vi "G#Debugger_CloneUI.vi"(1 "RootClass":string) -> ()   [LabVIEW 2017, in "G#Debugger.lvlib"]
doc: "Debugger for G# Objects."
uses:
  <vilib>/addons/_AddQ/G#Debugger/G#Debugger.lvlib
  <vilib>/addons/_AddQ/G#Debugger/private/G#Debugger_SubPanelInfo.ctl
  <vilib>/addons/_AddQ/G#Object/G#Object.lvclass
  <vilib>/addons/_AddQ/G#Object/utils/G#Object_ClassHierarchy.ctl
  <vilib>/addons/_AddQ/G#Debugger/private/G#Debugger_TreeElement.ctl
  <vilib>/addons/_AddQ/G#Debugger/private/G#Debugger_DebugDialog.vi
  <vilib>/Platform/browser.llb/Open URL in Default Browser (string).vi
panel:
  in  "AggregatorsTags":i32(listbox)
  in  "Help":bool
  out "Application Instance":string
  in  "Window Behaviour":bool
  in  "Window Transparency":u8(slide) max=75 scale=0.0..75.0
  in  "External Create Process Running":bool
  in  "Tab Control":enum32{"Objects", "Trace", "Active Debug"}(tab)
  out "RootCls":string caption="Root Class"
  in  "Aggregators":i32(listbox)
  in  "AggregatesTags":i32(listbox)
  in  "Aggregates":i32(listbox)
  in  "Highlight Aggregates?":bool=TRUE
  in  "Attributes":bool
  in  "Inheritance":i32(listbox)
  in  "Destroy":bool
  in  "ObjectTree":string(tree) caption="Object Tree"
  in  "Refresh":bool
  out "# of Users":i32
  out "Counter":bool
  out "Object Name":string
  out "Full Class Name":string
  in  "Poll Time (ms)":i32=200 min=0
  in  "Garbage collect":bool
  out "Object ID":u32 format="%x"
  in  "Hide Empty Classes?":bool=TRUE
  out "Owner":string
  out "Connected?":bool
  in  "ShowAggregators":bool
  out "To String":string
  in  "Filter Expression":string
  in  "Trace Direction":bool=TRUE
  in  "Clear":bool
  in  "Save":bool
  out "Trace":string
  in  "Max Lines":u32=1000
  out "Run State":string
  out "CachedObjId":u32 caption="Object ID" format="%x"
  in  "Abort VI":bool
  in  "Run VI":bool
  in  "Open Panel":bool
  in  "DebugTree":string(tree)
  in  "Enable Active Debug":bool
  out "Icon":picture
  out "Cached Ref Valid":bool
  in  "Wait Until Done":bool=TRUE
  out "Cached Reference Class Name":string
  out "G# Version":string
  # "G# Clone Debugger"
  # "< Poll to update >"
  # "These logs will also always appear in the NI LabVIEW Desktop Execution Trace, even without debugger running."
  # "The last created reference is automatically cashed and copied to all the new selected , opened or executed methods 'reference in'."
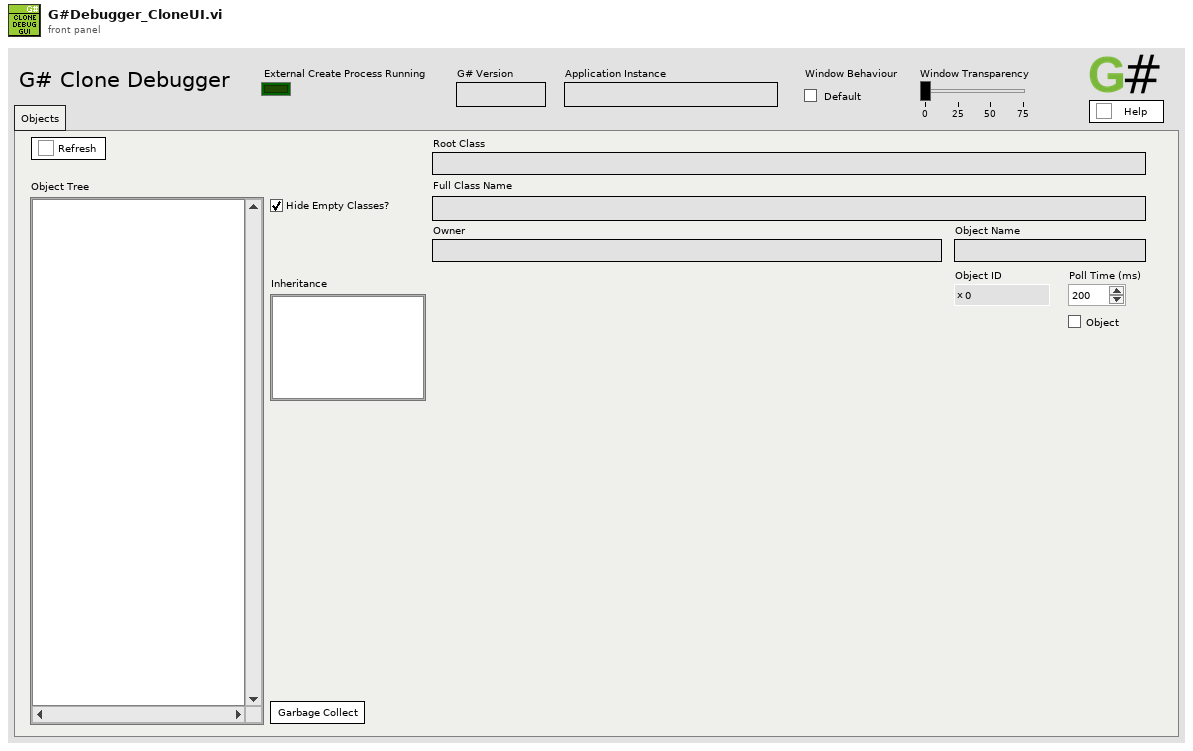
[diagram p1: front panel]
types:
  T1 = cluster{"ObjectName":string, "ObjectID":u32, "Users":i32, "Counter":bool, "AttributeRefs":u32[], "FullClassName":string, "ClassName":string, "Create method":enum16{"Create", "Create or look up existing", "Look up existing"}, "GenericDestructorExists":bool, "Owner":string}[]
  T2 = cluster{"Path":path, "ClsNames":string[], "ClsPaths":path[], "ParPaths":path[]}
  T3 = cluster{"ClassInfoDvr":refnum<data-value>, "sub panel dvr":refnum<data-value>, "CloneUIevent":refnum<user-event>, "Active Project":refnum<vi>, "Front Panel":refnum<vi>}
  T4 = typedef "G#Debugger.lvlib/G#Debugger_SubPanelInfo.ctl" = cluster{"Ref":refnum<class "G#Object.lvclass">, "class hierarchy":T5[], "class attributes":path[], "object attributes":path[], "inheritance index":i32, "is class attributes":bool, "vi reference":refnum<vi>}
  T5 = typedef "G#Object.lvclass/G#Object_ClassHierarchy.ctl" = cluster{"ClassName":string, "FullClassName":string, "ClassPath":path, "IsLeaf":bool}
  T6 = enum8{"Enabled", "Disabled", "Disabled and Grayed Out"}
  T7 = typedef "G#Debugger.lvlib/G#Debugger_TreeElement.ctl" = cluster{"Name":string, "Tag":string, "ParentTag":string, "Position":i32}
  T8 = cluster{"ObjectTree":string, "Attributes":bool, "Inheritance":i32}
  T9 = cluster{"Active Item Row Number":i32, "name":string}
  T10 = enum32{"Invalid", "Default", "Floating", "Floating/Auto-Hide", "Modal"}
  T11 = cluster{"ObjectName":string, "ObjectID":u32, "Users":i32, "Counter":bool, "AttributeRefs":u32[], "FullClassName":string, "ClassName":string, "Create method":enum16{"Create", "Create or look up existing", "Look up existing"}, "GenericDestructorExists":bool, "Owner":string}
  T12 = cluster{"ObjectTree":string, bool, "Inheritance":i32}
  T13 = enum32{"Bad", "Idle", "Run top level", "Running"}
  T14 = cluster{"Active Item Row Number":i32, "name":string}[]
  T15 = typedef "imagedata.ctl" = cluster{"image type":i32, "image depth":i32, "image":u8[], "mask":u8[], "colors":u32[], "Rectangle":cluster{"left":i16, "top":i16, "right":i16, "bottom":i16}}
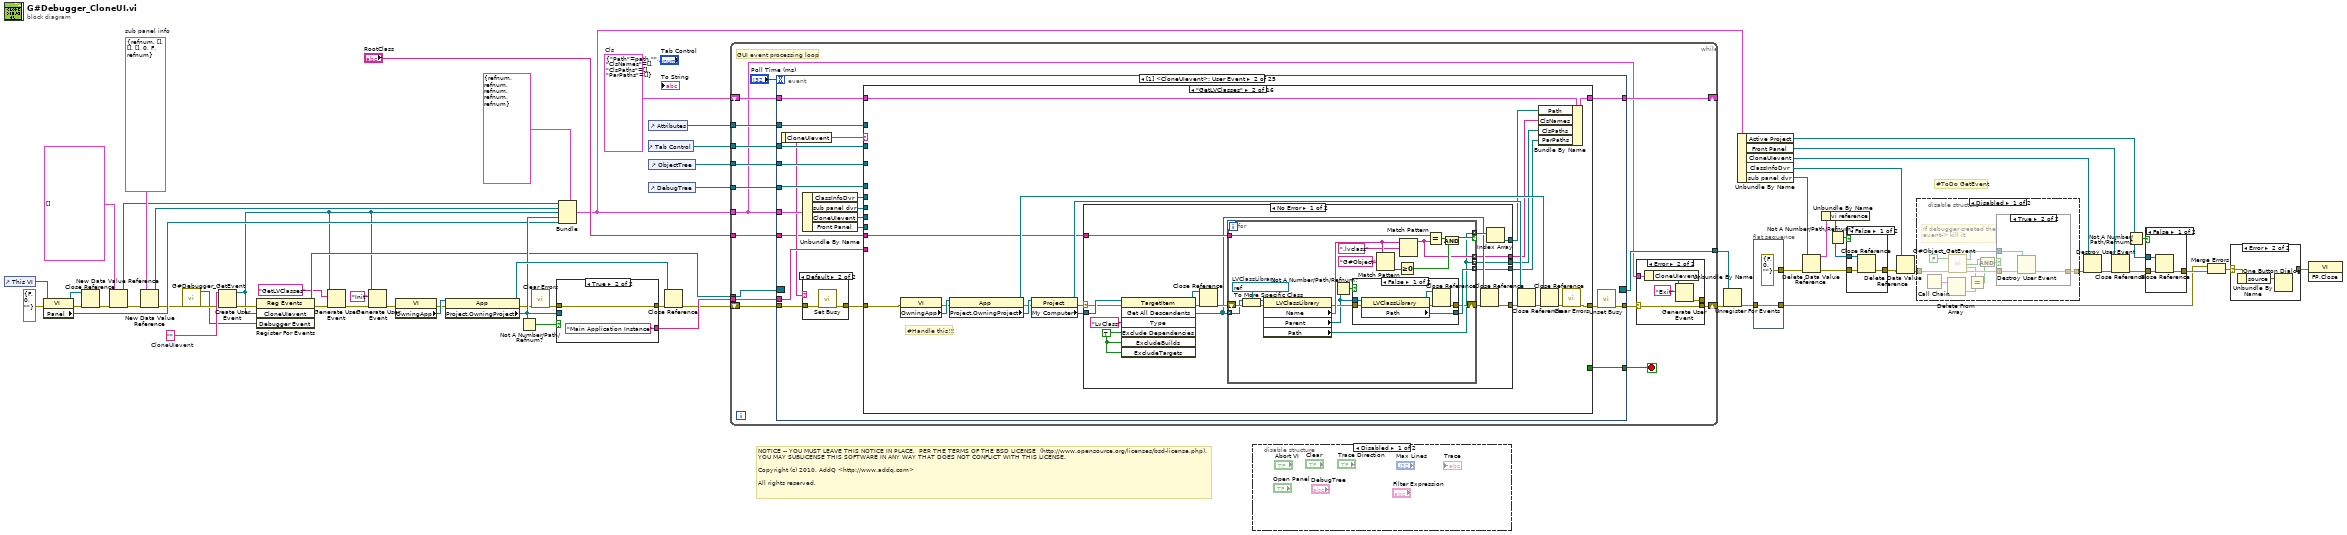
[diagram p0: block diagram]
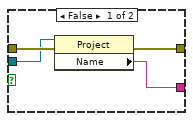
[diagram p7: hidden frame]
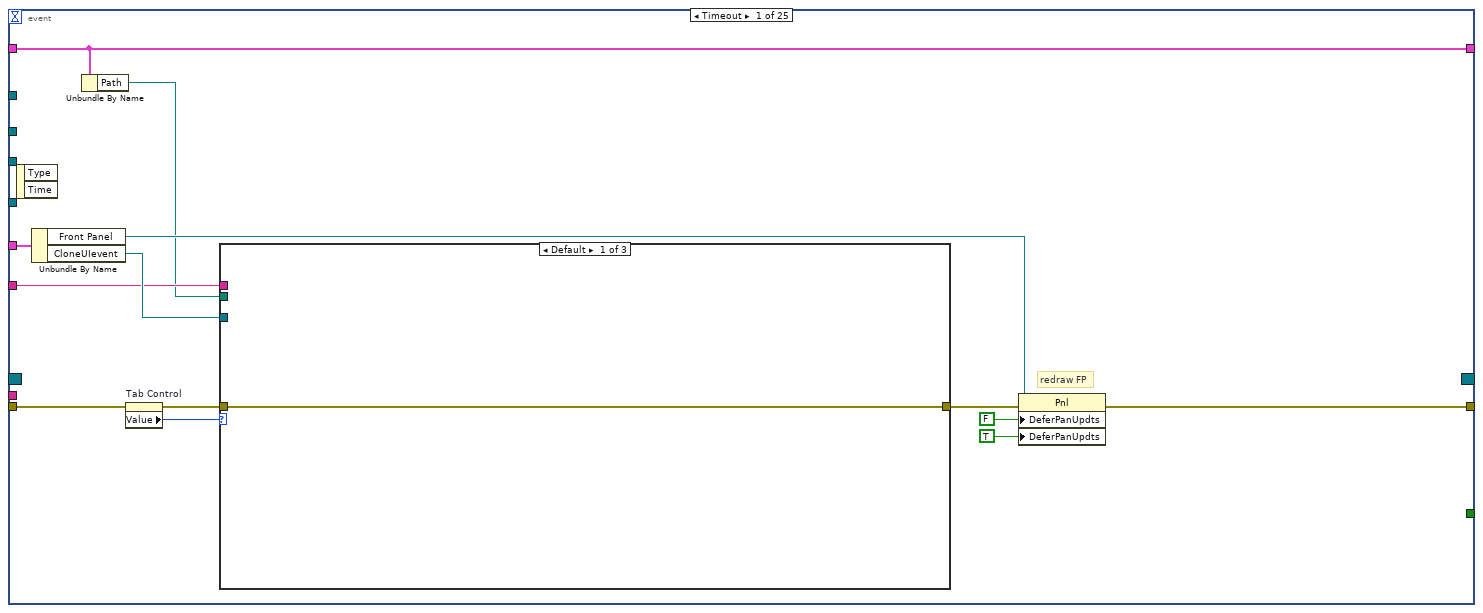
[diagram p10: hidden frame]
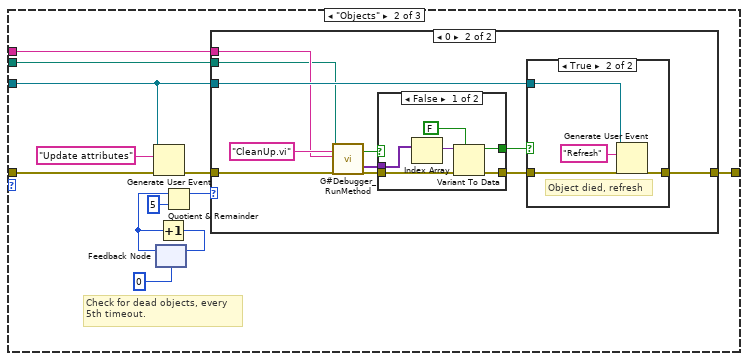
[diagram p11: hidden frame]
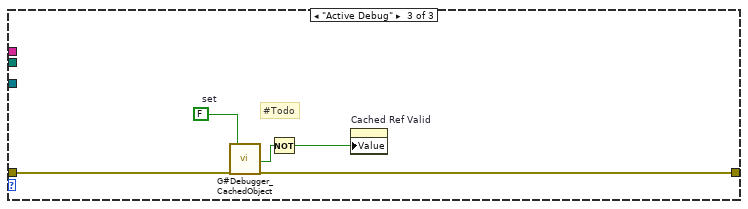
[diagram p15: hidden frame]
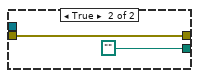
[diagram p18: hidden frame]
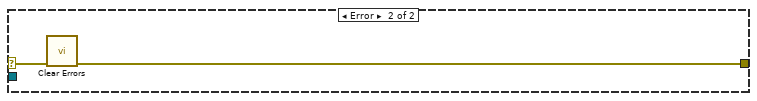
[diagram p19: hidden frame]
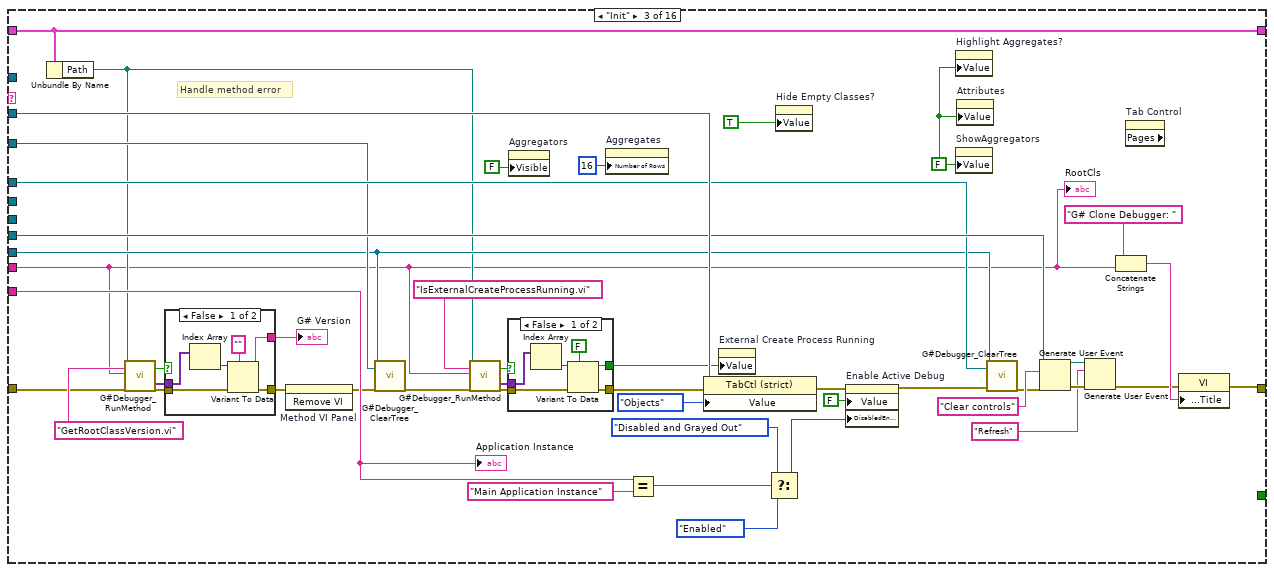
[diagram p20: hidden frame]
diagram:
  w6 = T2 {"Path"=path "", "ClsNames"=[], "ClsPaths"=[], "ParPaths"=[]}  # Cls
  w35 = ""  # CloneUIevent
  w55 = T4 {"Ref"=refnum, "class hierarchy"=[], "class attributes"=[], "object attributes"=[], "inheritance index"=0, "is class attributes"=FALSE, "vi reference"=refnum}  # sub panel info
  # "#ToDo GetEvent"
  # "NOTICE -- YOU MUST LEAVE THIS NOTICE IN PLACE.  PER THE TERMS OF THE BSD LICENSE  (http://www.opensource.org/licenses/bsd-license.php).\nYOU MAY SUBLICENSE THIS SOFTWARE IN ANY WAY THAT DOES NOT CONFLICT WITH THIS LICENSE.\n\nCopyright (c) 2010, AddQ <http://www.addq.com>\n\nAll rights reserved."
  n1 = control-ref of="This VI"() -> (w40:refnum<vi>)
  n2 = property class="VI"(reference=w40, error in=errorcluster {"status"=FALSE, "code"=0, "source"=""} ("error in (no error)")) -> (reference out=w43:refnum<vi>, error out=w44:errorcluster, "Panel"=w42:refnum<vi>)
  n3 = Close Reference(reference=w43, error in (no error)=w44) -> (error out=w41:errorcluster)
  n4 = New Data Value Reference(data value=T1 [], error in=w41) -> (data value reference=w3:refnum<data-value>, error out=w56:errorcluster)
  n5 = New Data Value Reference(data value=w55, error in=w56) -> (data value reference=w54:refnum<data-value>, error out=w34:errorcluster)
  n6 = call <vilib>:"G#Debugger_GetEvent.vi"("error in (no error)"=w34) -> ("Debugger Event"=w32:refnum<user-event>, "error out"=w33:errorcluster)  [unwired: 17 in]
  n7 = Create User Event(user event datatype=w35, error in=w33) -> (user event=w9:refnum<user-event>, error out=w36:errorcluster)
  n8 = register-events(error in=w36, w9, w32) -> (reference out=w39:refnum<event-registration>, error out=w8:errorcluster)  [unwired: 1 in]
  n9 = Generate User Event(user event=w9, event data cluster="GetLVClasses" ("event data"), error in=w8) -> (error out=w7:errorcluster)  [unwired: 1 in, 1 out]
  n10 = Generate User Event(user event=w9, event data cluster="Init" ("event data"), error in=w7) -> (error out=w52:errorcluster)  [unwired: 1 in, 1 out]
  n11 = property class="VI"(error in=w52) -> (error out=w51:errorcluster, "OwningApp"=w53:refnum<vi>)  [unwired: 1 in, 1 out]
  n12 = property class="App"(reference=w53, error in=w51) -> (reference out=w48:refnum<vi>, error out=w46:errorcluster, "Project.OwningProject"=w47:refnum<vi>)
  n13 = Not A Number/Path/Refnum?(number/path/refnum=w47) -> (NaN/Path/Refnum?=w50:bool)
  n14 = call <vilib>:"Clear Errors.vi"("error in (no error)"=w46) -> ("error out"=w45:errorcluster)  [unwired: 5 in, 1 out]
  n15 = case shown="True" w50 {
    tunnel: w45 -> [w68 w70]
    tunnel: w47 -> [w67 _]
    tunnel: [w65 w70] -> w49
    tunnel: [w66 "Main Application Instance" ("Name")] -> w38
    frame False {
      n16 = property class="Project"(reference=w67, error in=w68) -> (error out=w65:errorcluster, "Name"=w66:string)  [unwired: 1 out]
    }
    frame True {
    }
  }
  n17 = Bundle(cluster=T3 {"ClassInfoDvr"=refnum, "sub panel dvr"=refnum, "CloneUIevent"=refnum, "Active Project"=refnum, "Front Panel"=refnum} ("refs"), "ClassInfoDvr"=w3, "sub panel dvr"=w54, "CloneUIevent"=w9, "Active Project"=w47, "Front Panel"=w42) -> (w14:T3)
  n18 = control-ref of="Attributes"() -> (w59:refnum<vi>)
  n19 = control-ref of="Tab Control"() -> (w64:refnum<vi>)
  n20 = control-ref of="ObjectTree"() -> (w60:refnum<vi>)
  n21 = control-ref of="DebugTree"() -> (w63:refnum<vi>)
  n22 = Close Reference(reference=w48, error in (no error)=w49) -> (error out=w37:errorcluster)
  n23 = while {
    shift-right: [w73] -> w62
    shift-left: w37 -> [w82]
    tunnel: w60 -> [w86]
    tunnel: w14 -> [w71]
    tunnel: w64 -> [w84]
    tunnel: w63 -> [w83]
    tunnel: w39 -> [w81]
    tunnel: [w78] -> w61
    tunnel: w38 -> [w79]
    tunnel: w59 -> [w77]
    tunnel: "RootClass" -> [w76]
    shift-right: [w75] -> _
    shift-left: w6 -> [w74]
    stop <- w85 stop-if-true
    # "GUI event processing loop"
    n24 = event shown="[1] <CloneUIevent>: User Event" {
      selector: w81 -> [_ _ _ _ _ _ _ _ _ _ _ _ _ _ _ _ _ _ _ _ _ _ _ _ _]
      dyn-events: [_ _ _ _ _ _ _ _ _ _ _ _ _ _ _ _ _ _ _ _ _ _ _ _ _] -> w78
      timeout: "Poll Time (ms)" -> [_ _ _ _ _ _ _ _ _ _ _ _ _ _ _ _ _ _ _ _ _ _ _ _ _]
      tunnel: w82 -> [w101 w153 w883 w894 w902 w913 w928 w933 w986 w1041 w1063 w1071 w1076 w1084 w1089 w1102 w1131 w1166 w1172 w1222 w1230 w1236 w1250 w1266 w1277]
      tunnel: [w98 w155 w882 w894 w902 w912 w927 w932 w981 w1040 w1062 w1072 w1074 w1082 w1095 w1114 w1129 w1163 w1171 w1221 w1229 w1235 w1250 w1265 w1274] -> w72
      tunnel: w86 -> [_ w166 _ w895 w903 _ _ _ w985 _ _ w1070 _ _ _ _ w1128 _ _ _ _ _ _ _ w1276]
      tunnel: [_ w165 _ _ _ _ FALSE _ _ _ _ _ _ _ _ _ _ _ _ _ _ _ _ _ _] -> w85
      tunnel: w71 -> [w105 w164 w881 _ _ w911 w926 w931 w983 _ w1061 _ w1075 w1083 _ w1112 w1125 _ w1170 _ _ _ _ _ w1273]
      tunnel: w84 -> [_ w161 _ _ _ _ _ _ _ _ _ _ _ _ _ _ _ _ _ _ _ _ _ _ _]
      tunnel: w83 -> [_ w159 _ _ _ _ _ _ _ _ _ _ _ _ _ _ _ _ w1173 _ _ _ _ _ _]
      tunnel: w79 -> [_ w158 _ _ _ _ _ _ _ _ _ _ _ _ _ _ _ _ w1169 _ _ _ _ _ _]
      tunnel: w77 -> [_ w151 _ _ _ _ _ _ _ _ _ _ _ _ _ _ _ _ _ _ _ _ _ _ _]
      tunnel: w76 -> [w95 w150 _ _ _ _ _ _ _ _ _ _ _ _ w1090 w1098 _ _ _ _ _ w1233 _ w1262 _]
      tunnel: [w94 w149 w880 w891 w899 w907 w921 w929 w969 w1030 w1060 w1066 w1073 w1079 w1087 w1106 w1124 w1162 w1167 w1218 w1224 w1232 w1247 w1264 w1272] -> w75
      tunnel: w74 -> [w94 w148 w880 w891 w899 w907 w921 w929 w969 w1030 w1060 w1066 w1073 w1079 w1087 w1106 w1124 w1162 w1167 w1218 w1224 w1232 w1247 w1264 w1272]
      event Timeout {
        # "redraw FP"
        n25 = event-data() -> ()  [unwired: 1 in, 2 out]
        n26 = Unbundle By Name(w105) -> ("Front Panel"=w99:refnum<vi>, "CloneUIevent"=w104:refnum<user-event>)
        n27 = Unbundle By Name(w94) -> ("Path"=w93:path)
        n28 = property on="Tab Control" class="TabCtl (strict)"(error in=w101) -> (error out=w102:errorcluster, "Value"=w103:enum32{"Objects", "Trace", "Active Debug"})  [unwired: 1 in, 1 out]
        n29 = case shown="Default" w103 {
          tunnel: w102 -> [w106 w118 w145]
          tunnel: w104 -> [_ w114 _]
          tunnel: [w106 w115 w144] -> w100
          tunnel: w93 -> [_ w108 _]
          tunnel: w95 -> [_ w107 _]
          frame Default {
          }
          frame "Objects" {
            # "Check for dead objects, every\n5th timeout."
            n30 = Generate User Event(user event=w114, event data cluster="Update attributes" ("event data"), error in=w118) -> (error out=w116:errorcluster)  [unwired: 1 in, 1 out]
            n31 = feedback #1(u64 0) -> (w110:u64)
            n32 = Increment(x=w110) -> (x+1=w109:u64)
            n33 = feedback-in #1(w109) -> ()
            n34 = Quotient & Remainder(x=w110, y=u64 5) -> (x-y*floor(x/y)=w113:u64)  [unwired: 1 out]
            n35 = case shown="0" w113 {
              tunnel: w116 -> [w119 w127]
              tunnel: [w119 w130] -> w115
              tunnel: w114 -> [_ w129]
              tunnel: w108 -> [_ w121]
              tunnel: w107 -> [_ w126]
              frame Default {
              }
              frame 0 {
                n36 = call <vilib>:"G#Debugger_RunMethod.vi"("ClassPath"=w121, "MethodName"="CleanUp.vi" ("name or relative path"), "ClassPrefix"=w126, "error in (no error)"=w127) -> ("Error?"=w120:bool, "ControlValue out"=w125:variant[], "error out"=w124:errorcluster)  [unwired: 13 in]
                n37 = case shown="False" w120 {
                  tunnel: w125 -> [w136 _]
                  tunnel: w124 -> [w135 w137]
                  tunnel: [w132 _] -> w123
                  tunnel: [w131 w137] -> w122
                  frame False {
                    n38 = Index Array(array=w136) -> (element=w133:variant)  [unwired: 1 in]
                    n39 = Variant To Data(error in=w135, type=FALSE, Variant=w133) -> (data=w132:bool, error out=w131:errorcluster)
                  }
                  frame True {
                  }
                }
                n40 = case shown="True" w123 {
                  tunnel: w122 -> [w138 w141]
                  tunnel: [w138 w140] -> w130
                  tunnel: w129 -> [_ w139]
                  frame False {
                  }
                  frame True {
                    # "Object died, refresh"
                    n41 = Generate User Event(user event=w139, event data cluster="Refresh" ("event data"), error in=w141) -> (error out=w140:errorcluster)  [unwired: 1 in, 1 out]
                  }
                }
              }
            }
          }
          frame "Active Debug" {
            w147 = FALSE  # set
            # "#Todo"
            n42 = call <vilib>:"G#Debugger_CachedObject.vi"("error in (no error)"=w145, "set"=w147) -> ("not a refnum?"=w146:bool, "error out"=w144:errorcluster)  [unwired: 15 in, 1 out]
            n43 = Not(x=w146) -> (.not. x?=w143:bool)
            n44 = property on="Cached Ref Valid" class="Bool (strict)"("Value"=w143) -> ()  [unwired: 2 in, 2 out]
          }
        }
        n45 = property class="Pnl"(reference=w99, error in=w100, "DeferPanUpdts"=FALSE ("Defer Panel Updates"), "DeferPanUpdts"=TRUE ("Defer Panel Updates")) -> (error out=w98:errorcluster)  [unwired: 1 out]
      }
      event User Event {
        n46 = event-data() -> ("CloneUIevent"=w154:string)  [unwired: 1 in]
        n47 = Unbundle By Name(w164) -> ("ClassInfoDvr"=w163:refnum<data-value>, "sub panel dvr"=w162:refnum<data-value>, "CloneUIevent"=w160:refnum<user-event>, "Front Panel"=w157:refnum<vi>)
        n48 = case shown="Default" w154 {
          tunnel: w153 -> [w167 w169]
          tunnel: [w167 w168] -> w152
          frame "Clear object tab", "Update attributes" {
          }
          frame Default {
            n49 = call <vilib>:"Set Busy.vi"("error in (no error)"=w169) -> ("error out"=w168:errorcluster)  [unwired: 9 in, 1 out]
          }
        }
        n50 = case shown="\"GetLVClasses\"" w154 {
          selector: w154 -> [_ _ _ _ _ _ _ _ _ _ _ _ w708 _ _ w878]
          tunnel: [w171 w178 w258 w301 w312 w322 w347 w374 w439 w463 w606 w655 w704 w712 w764 w879] -> w156
          tunnel: w152 -> [w171 w180 w250 w302 w312 w321 w337 w376 w441 w458 w609 w656 w704 w716 w768 w879]
          tunnel: [_ _ _ _ _ TRUE _ _ _ _ _ _ _ _ _ _] -> w165
          tunnel: w163 -> [_ _ _ _ _ _ _ w380 w430 w466 _ _ _ w714 w766 _]
          tunnel: w166 -> [_ _ w276 _ _ _ _ w391 w440 w460 w610 _ _ w711 w763 _]
          tunnel: w162 -> [_ _ _ _ _ _ _ _ _ w465 w598 _ _ _ _ _]
          tunnel: w161 -> [_ _ w283 _ _ _ _ _ _ _ _ _ _ _ _ _]
          tunnel: w160 -> [_ _ w281 w300 _ _ w349 w384 w438 w464 _ _ _ _ _ _]
          tunnel: w159 -> [_ _ w277 _ _ _ _ _ _ _ _ _ _ _ _ _]
          tunnel: w158 -> [_ _ w274 _ _ _ _ _ _ _ _ _ _ _ _ _]
          tunnel: w157 -> [_ _ w263 _ _ _ _ w392 w436 _ _ _ _ w710 w762 _]
          tunnel: w151 -> [_ _ _ _ _ _ _ _ _ w461 _ _ _ _ _ _]
          tunnel: w150 -> [_ w179 w239 _ _ w318 w339 w370 w429 _ w604 _ _ _ _ _]
          tunnel: [w170 w172 w245 w298 w307 w317 w350 w383 w427 w459 w612 w654 w703 w709 w761 w875] -> w149
          tunnel: w148 -> [w170 w177 w245 w298 w307 w317 w350 w383 w427 w459 w612 w654 w703 w709 w761 w875]
          frame Default {
          }
          frame "GetLVClasses" {
            # "#Handle this!!!"
            n51 = property class="VI"(error in=w180) -> (error out=w190:errorcluster, "OwningApp"=w191:refnum<vi>)  [unwired: 1 in, 1 out]
            n52 = property class="App"(reference=w191, error in=w190) -> (reference out=w189:refnum<vi>, error out=w183:errorcluster, "Project.OwningProject"=w184:refnum<vi>)
            n53 = property class="Project"(reference=w184, error in=w183) -> (reference out=w188:refnum<vi>, error out=w186:errorcluster, "My Computer"=w187:refnum<vi>)
            n54 = case shown="No Error" w186 {
              selector: w186 -> [w201 w237]
              tunnel: w187 -> [w205 _]
              tunnel: [w199 w236] -> w185
              tunnel: w179 -> [w198 _]
              tunnel: [w196 _] -> w176
              tunnel: [w194 _] -> w173
              tunnel: [w193 _] -> w175
              tunnel: [w192 _] -> w174
              frame No Error {
                w206 = TRUE ("ExcludeDependencies")
                n55 = invoke class="TargetItem" method="Get All Descendents"(reference=w205, error in=w201, "Type"="LvClass", "Exclude Dependencies"=w206, "ExcludeBuilds"=w206, "ExcludeTargets"=w206) -> (reference out=w204:refnum<vi>, error out=w202:errorcluster, "All Descendents"=w195:refnum<vi>[])  [unwired: 1 in, 4 out]
                n56 = Close Reference(reference=w204, error in (no error)=w202) -> (error out=w203:errorcluster)
                n57 = for {
                  tunnel: w195 -> [w220] mode=indexing
                  shift-right: [w211] -> w200
                  shift-left: w203 -> [w227]
                  tunnel: w198 -> [w219]
                  tunnel: [w210] -> w197 mode=indexing if=w215
                  tunnel: [w210] -> w192 mode=indexing
                  tunnel: [w214] -> w193 mode=indexing
                  tunnel: [w212] -> w194 mode=indexing
                  w226 = refnum<vi> refnum  # LVClassLibrary
                  n58 = To More Specific Class(target class=w226, reference=w220, error in=w227) -> (specific class reference=w221:refnum<vi>, error out=w222:errorcluster)
                  n59 = property class="LVClassLibrary"(reference=w221, error in=w222) -> (error out=w213:errorcluster, "Name"=w225:string, "Parent"=w209:refnum<vi>, "Path"=w210:path)  [unwired: 1 out]
                  n60 = Not A Number/Path/Refnum?(number/path/refnum=w209) -> (NaN/Path/Refnum?=w208:bool)
                  n61 = case shown="False" w208 {
                    tunnel: w209 -> [w233 _]
                    tunnel: w213 -> [w232 w235]
                    tunnel: [w231 path ""] -> w212
                    tunnel: [w228 w235] -> w211
                    frame False {
                      n62 = property class="LVClassLibrary"(reference=w233, error in=w232) -> (reference out=w229:refnum<vi>, error out=w230:errorcluster, "Path"=w231:path)
                      n63 = Close Reference(reference=w229, error in (no error)=w230) -> (error out=w228:errorcluster)
                    }
                    frame True {
                    }
                  }
                  n64 = Match Pattern(string=w225, regular expression="G#Object" ("string")) -> (offset past match=w216:i32)  [unwired: 1 in, 3 out]
                  n65 = Greater Or Equal To 0?(x=w216) -> (x >= 0?=w218:bool)
                  n66 = Match Pattern(string=w225, regular expression=".lvclass") -> (before substring=w214:string)  [unwired: 1 in, 3 out]
                  n67 = Equal?(x=w219, y=w214) -> (x = y?=w217:bool)
                  n68 = And(x=w217, y=w218) -> (x .and. y?=w215:bool)
                }
                n69 = Close Reference(reference=w195, error in (no error)=w200) -> (error out=w199:errorcluster)
                n70 = Index Array(array=w197) -> (element=w196:path)  [unwired: 1 in]
              }
              frame Error {
                n71 = call <vilib>:"Clear Errors.vi"("error in (no error)"=w237) -> ("error out"=w236:errorcluster)  [unwired: 5 in, 1 out]
              }
            }
            n72 = Close Reference(reference=w188, error in (no error)=w185) -> (error out=w182:errorcluster)
            n73 = Bundle By Name(cluster=w177, "Path"=w176, "ClsNames"=w175, "ClsPaths"=w174, "ParPaths"=w173) -> (w172:T2)
            n74 = Close Reference(reference=w189, error in (no error)=w182) -> (error out=w181:errorcluster)
            n75 = call <vilib>:"Clear Errors.vi"("error in (no error)"=w181) -> ("error out"=w178:errorcluster)  [unwired: 5 in, 1 out]
          }
          frame "Init" {
            w240 = FALSE ("ShowAggregators")
            # "Handle method error"
            n76 = Unbundle By Name(w245) -> ("Path"=w244:path)
            n77 = call <vilib>:"G#Debugger_RunMethod.vi"("ClassPath"=w244, "MethodName"="GetRootClassVersion.vi", "ClassPrefix"=w239, "error in (no error)"=w250) -> ("Error?"=w242:bool, "ControlValue out"=w247:variant[], "error out"=w248:errorcluster)  [unwired: 13 in]
            n78 = case shown="False" w242 {
              tunnel: [w287 w290] -> w252
              tunnel: [w286 _] -> w249
              tunnel: w248 -> [w285 w290]
              tunnel: w247 -> [w284 _]
              frame False {
                n79 = Index Array(array=w284) -> (element=w289:variant)  [unwired: 1 in]
                n80 = Variant To Data(error in=w285, type="", Variant=w289) -> (data=w286:string, error out=w287:errorcluster)
              }
              frame True {
              }
            }
            "G# Version" <- w249
            n81 = invoke on="Method VI Panel" class="SubPanel" method="Remove VI"(error in=w252) -> (error out=w268:errorcluster)  [unwired: 2 in, 2 out]
            n82 = call <vilib>:"G#Debugger_ClearTree.vi"("Front Panel"=w263, "Tree"=w276, "error in (no error)"=w268) -> ("error out"=w253:errorcluster)  [unwired: 16 in]
            n83 = call <vilib>:"G#Debugger_RunMethod.vi"("ClassPath"=w244, "MethodName"="IsExternalCreateProcessRunning.vi", "ClassPrefix"=w239, "error in (no error)"=w253) -> ("Error?"=w243:bool, "ControlValue out"=w246:variant[], "error out"=w254:errorcluster)  [unwired: 13 in]
            n84 = case shown="False" w243 {
              tunnel: [w295 _] -> w256
              tunnel: [w294 w297] -> w255
              tunnel: w254 -> [w292 w297]
              tunnel: w246 -> [w291 _]
              frame False {
                n85 = Index Array(array=w291) -> (element=w293:variant)  [unwired: 1 in]
                n86 = Variant To Data(error in=w292, type=FALSE, Variant=w293) -> (data=w295:bool, error out=w294:errorcluster)
              }
              frame True {
              }
            }
            n87 = property on="Aggregators" class="LstBox (strict)"("Visible"=FALSE) -> ()  [unwired: 2 in, 2 out]
            n88 = property on="Aggregates" class="LstBox (strict)"("Number of Rows"=u32 16) -> ()  [unwired: 2 in, 2 out]
            n89 = Equal?(x=w274, y="Main Application Instance") -> (x = y?=w272:bool)
            n90 = property class="TabCtl (strict)"(reference=w283, error in=w255, "Value"=enum32{"Objects", "Trace", "Active Debug"}."Objects") -> (error out=w280:errorcluster)  [unwired: 1 out]
            n91 = property on="External Create Process Running" class="Bool (strict)"("Value"=w256) -> ()  [unwired: 2 in, 2 out]
            n92 = Select(t=T6."Disabled and Grayed Out" ("Disabled"), s=w272, f=T6."Enabled" ("Disabled")) -> (s? t:f=w269:T6)
            n93 = property on="Hide Empty Classes?" class="Bool (strict)"("Value"=TRUE ("Highlight Aggregates?")) -> ()  [unwired: 2 in, 2 out]
            n94 = property on="Enable Active Debug" class="Bool (strict)"(error in=w280, "Value"=FALSE ("Enable Active Debug"), "DisabledEnum"=w269) -> (error out=w267:errorcluster)  [unwired: 1 in, 1 out]
            n95 = property on="Highlight Aggregates?" class="Bool (strict)"("Value"=w240) -> ()  [unwired: 2 in, 2 out]
            n96 = property on="ShowAggregators" class="Bool (strict)"("Value"=w240) -> ()  [unwired: 2 in, 2 out]
            n97 = property on="Attributes" class="Bool (strict)"("Value"=w240) -> ()  [unwired: 2 in, 2 out]
            n98 = call <vilib>:"G#Debugger_ClearTree.vi"("Front Panel"=w263, "Tree"=w277, "error in (no error)"=w267) -> ("error out"=w275:errorcluster)  [unwired: 16 in]
            n99 = Generate User Event(user event=w281, event data cluster="Clear controls" ("event data"), error in=w275) -> (user event out=w266:refnum<user-event>, error out=w265:errorcluster)  [unwired: 1 in]
            n100 = Generate User Event(user event=w266, event data cluster="Refresh" ("event data"), error in=w265) -> (error out=w238:errorcluster)  [unwired: 1 in, 1 out]
            n101 = Concatenate Strings("G# Clone Debugger: ", w239) -> (w259:string)
            n102 = property on="Tab Control" class="TabCtl (strict)" props=["Pages"]() -> ()  [unwired: 2 in, 3 out]
            n103 = property class="VI"(error in=w238, "Front Panel.Title"=w259) -> (error out=w258:errorcluster)  [unwired: 1 in, 1 out]
            "Application Instance" <- w274
            "RootCls" <- w239
          }
          frame "Clear controls" {
            w303 = ""
            n104 = property on="Cached Ref Valid" class="Bool (strict)"("Value"=FALSE ("Counter")) -> ()  [unwired: 2 in, 2 out]
            n105 = property on="Run State" class="Str"("Value"=w303) -> ()  [unwired: 2 in, 2 out]
            n106 = call "Empty Picture"() -> ("empty picture"=w305:picture)
            n107 = property on="Trace" class="Str"("Value"=w303) -> ()  [unwired: 2 in, 2 out]
            n108 = property on="Icon" class="Pict"("Value"=w305) -> ()  [unwired: 2 in, 2 out]
            n109 = property on="Cached Reference Class Name" class="Str"("Value"=w303) -> ()  [unwired: 2 in, 2 out]
            n110 = property on="CachedObjId" class="DigNum (strict)"("Value"=u32 0 ("Object ID")) -> ()  [unwired: 2 in, 2 out]
            n111 = Generate User Event(user event=w300, event data cluster="Clear object tab" ("event data"), error in=w302) -> (error out=w301:errorcluster)  [unwired: 1 in, 1 out]
          }
          frame "Clear object tab" {
            w308 = 0 ("Top Row")
            w309 = string[] [] ("Item Names")
            w310 = -1 ("Inheritance")
            w311 = ""
            n112 = property on="Object Name" class="Str"("Value"=w311) -> ()  [unwired: 2 in, 2 out]
            n113 = property on="Owner" class="Str"("Value"=w311) -> ()  [unwired: 2 in, 2 out]
            n114 = property on="Full Class Name" class="Str"("Value"=w311) -> ()  [unwired: 2 in, 2 out]
            n115 = property on="# of Users" class="DigNum (strict)"("Value"=0 ("Nr of Users")) -> ()  [unwired: 2 in, 2 out]
            n116 = property on="Object ID" class="DigNum (strict)"("Value"=u32 0 ("Object ID")) -> ()  [unwired: 2 in, 2 out]
            n117 = property on="Counter" class="Bool (strict)"("Value"=FALSE ("Counter")) -> ()  [unwired: 2 in, 2 out]
            n118 = property on="Inheritance" class="LstBox (strict)"("Value"=w310, "Item Names"=w309, "Top Row"=w308) -> ()  [unwired: 2 in, 2 out]
            n119 = property on="Aggregates" class="LstBox (strict)"("Value"=w310, "Item Names"=w309, "Top Row"=w308) -> ()  [unwired: 2 in, 2 out]
            n120 = property on="Aggregators" class="LstBox (strict)"("Value"=w310, "Item Names"=w309, "Top Row"=w308) -> ()  [unwired: 2 in, 2 out]
          }
          frame "Exit" {
            n121 = property on="Enable Active Debug" class="Bool (strict)"(error in=w321) -> (error out=w320:errorcluster, "Value"=w319:bool)  [unwired: 1 in, 1 out]
            n122 = Unbundle By Name(w317) -> ("Path"=w316:path)
            n123 = case shown="True" w319 {
              tunnel: [w324 w331] -> w322
              tunnel: w320 -> [w324 w332]
              tunnel: w318 -> [_ w328]
              tunnel: w316 -> [_ w330]
              tunnel: [_ w329] -> _
              frame False {
              }
              frame True {
                n124 = To Variant(anything=TRUE) -> (Variant=w326:variant)
                n125 = Build Array(w326) -> (w325:variant[])
                n126 = call <vilib>:"G#Debugger_RunMethod.vi"("ClassPath"=w330, "MethodName"="GarbageCollector.vi", "ClassPrefix"=w328, "error in (no error)"=w332, "ControlValue"=w325) -> ("Error?"=w329:bool, "error out"=w331:errorcluster)  [unwired: 12 in, 1 out]
              }
            }
          }
          frame "Refresh" {
            n127 = Unbundle By Name(w350) -> ("Path"=w341:path)
            n128 = call <vilib>:"G#Debugger_RunMethod.vi"("ClassPath"=w341, "MethodName"="IsExternalCreateProcessRunning.vi", "ClassPrefix"=w339, "error in (no error)"=w337) -> ("Error?"=w343:bool, "ControlValue out"=w344:variant[], "error out"=w345:errorcluster)  [unwired: 13 in]
            n129 = case shown="False" w343 {
              tunnel: [w357 _] -> w342
              tunnel: [w356 w359] -> w338
              tunnel: w345 -> [w354 w359]
              tunnel: w344 -> [w353 _]
              frame False {
                n130 = Index Array(array=w353) -> (element=w355:variant)  [unwired: 1 in]
                n131 = Variant To Data(error in=w354, type=FALSE, Variant=w355) -> (data=w357:bool, error out=w356:errorcluster)
              }
              frame True {
              }
            }
            n132 = property on="External Create Process Running" class="Bool (strict)"(error in=w338, "Value"=w342) -> (error out=w336:errorcluster)  [unwired: 1 in, 1 out]
            n133 = property on="Highlight Aggregates?" class="Bool (strict)"() -> ("Value"=w352:bool)  [unwired: 2 in, 2 out]
            n134 = case shown="True" w352 {
              tunnel: [w365 w368] -> w334
              tunnel: w336 -> [w365 w367]
              tunnel: w349 -> [_ w366]
              frame False {
              }
              frame True {
                n135 = Generate User Event(user event=w366, event data cluster="Highlight aggregates" ("event data"), error in=w367) -> (error out=w368:errorcluster)  [unwired: 1 in, 1 out]
              }
            }
            n136 = property on="ShowAggregators" class="Bool (strict)"(error in=w334) -> (error out=w335:errorcluster, "Value"=w351:bool)  [unwired: 1 in, 1 out]
            n137 = case shown="True" w351 {
              tunnel: w335 -> [w360 w363]
              tunnel: [w360 w362] -> w346
              tunnel: w349 -> [_ w361]
              frame False {
              }
              frame True {
                n138 = Generate User Event(user event=w361, event data cluster="ListAggregators" ("event data"), error in=w363) -> (error out=w362:errorcluster)  [unwired: 1 in, 1 out]
              }
            }
            n139 = Generate User Event(user event=w349, event data cluster="UpdateTree" ("event data"), error in=w346) -> (error out=w347:errorcluster)  [unwired: 1 in, 1 out]
          }
          frame "UpdateTree" {
            n140 = Unbundle By Name(w383) -> ("ClsNames"=w382:string[], "Path"=w371:path)
            n141 = call <vilib>:"G#Debugger_RunMethod.vi"("ClassPath"=w371, "MethodName"="CleanUp.vi" ("name or relative path"), "ClassPrefix"=w370, "error in (no error)"=w376) -> ("error out"=w375:errorcluster)  [unwired: 13 in, 2 out]
            n142 = call <vilib>:"G#Debugger_RunMethod.vi"("ClassPath"=w371, "MethodName"="GetAllObjects.vi" ("name or relative path"), "ClassPrefix"=w370, "error in (no error)"=w375) -> ("Error?"=w381:bool, "ControlValue out"=w393:variant[], "error out"=w394:errorcluster)  [unwired: 13 in]
            n143 = case shown="False" w381 {
              tunnel: T1 [] -> [w404 w406]
              tunnel: [w403 w406] -> w377
              tunnel: w394 -> [w401 w405]
              tunnel: w393 -> [w400 _]
              tunnel: [w399 w405] -> w390
              frame False {
                n144 = Index Array(array=w400) -> (element=w402:variant)  [unwired: 1 in]
                n145 = Variant To Data(error in=w401, type=w404, Variant=w402) -> (data=w403:T1, error out=w399:errorcluster)
              }
              frame True {
              }
            }
            n146 = To Upper Case(1:w382) -> (0:w388:string[])
            n147 = for {
              tunnel: w377 -> [w425] mode=indexing
              tunnel: T7 {"Name"="", "Tag"="", "ParentTag"="", "Position"=0} ("TreeElement") -> [w418]
              tunnel: [w417] -> w378 mode=concatenating
              tunnel: w388 -> [w412]
              tunnel: [w413] -> w387 mode=indexing
              w422 = -1 ("Position")
              n148 = Unbundle By Name(w425) -> ("ClassName"=w416:string, "ObjectName"=w423:string, "ObjectID"=w420:u32)
              n149 = Number To Decimal String(number=w420) -> (decimal integer string=w421:string)  [unwired: 1 in]
              n150 = To Upper Case(1:w416) -> (0:w414:string)
              n151 = Search 1D Array(1D array=w412, element=w414) -> (index of element=w415:i32)  [unwired: 1 in]
              n152 = Bundle By Name(cluster=w418, "Name"=w423, "Tag"=w421, "ParentTag"=w416, "Position"=w422) -> (w419:T7)
              n153 = Bundle By Name(cluster=w418, "Name"=w416, "Tag"=w416, "Position"=w422) -> (w424:T7)
              n154 = Less Than 0?(x=w415) -> (x < 0?=w413:bool)
              n155 = Build Array(w424, w419) -> (w417:T7[])
            }
            n156 = call <vilib>:"G#Debugger_ClearTree.vi"("Front Panel"=w392, "Tree"=w391, "error in (no error)"=w390) -> ("error out"=w389:errorcluster)  [unwired: 16 in]
            n157 = Or Array Elements(Boolean array=w387) -> (logical OR=w386:bool)
            n158 = call <vilib>:"G#Debugger_AddObjectToTree.vi"("Front Panel"=w392, "Tree"=w391, "Elements"=w378, "error in (no error)"=w389) -> ("error out"=w385:errorcluster)  [unwired: 15 in]
            n159 = case shown="True" w386 {
              tunnel: w385 -> [w407 w411]
              tunnel: [w407 w410] -> w373
              tunnel: w384 -> [_ w409]
              frame False {
              }
              frame True {
                n160 = Generate User Event(user event=w409, event data cluster="GetLVClasses" ("event data"), error in=w411) -> (error out=w410:errorcluster)  [unwired: 1 in, 1 out]
              }
            }
            n161 = in-place {
              in-place-border: w377 -> [w398]
              n162 = in-place-dvr #2(w380) -> ()  [unwired: 2 out]
              n163 = in-place-dvr #2(w398) -> (w372:errorcluster)  [unwired: 1 out]
            }
            n164 = Merge Errors(w373, w372) -> (w374:errorcluster)
          }
          frame "Clear" {
            # "Clears tree and object cache"
            n165 = Unbundle By Name(w427) -> ("Path"=w426:path)
            n166 = call <vilib>:"G#Debugger_ClearTree.vi"("Front Panel"=w436, "Tree"=w440, "error in (no error)"=w441) -> ("error out"=w431:errorcluster)  [unwired: 16 in]
            n167 = in-place {
              in-place-border: w431 -> [w444]
              in-place-border: [w443] -> w433
              in-place-border: [w451] -> w434
              in-place-border: w426 -> [w442]
              in-place-border: w429 -> [w445]
              # "Remove\ndead objects"
              n168 = in-place-dvr #3(w430) -> (w450:T1, w451:errorcluster)
              n169 = Index Array(array=w450) -> (element=w449:T11)  [unwired: 1 in]
              n170 = call <vilib>:"G#Debugger_RunMethod.vi"("ClassPath"=w442, "MethodName"="CleanUp.vi" ("name or relative path"), "ClassPrefix"=w445, "error in (no error)"=w444) -> ("error out"=w443:errorcluster)  [unwired: 13 in, 2 out]
              n171 = Initialize Array(w449, 0 ("dimension size")) -> (w447:T1)
              n172 = in-place-dvr #3(w447) -> (w435:errorcluster)  [unwired: 1 out]
            }
            n173 = call <vilib>:"Clear Errors.vi"("error in (no error)"=w433) -> ("error out"=w432:errorcluster)  [unwired: 5 in, 1 out]
            n174 = Merge Errors(w435, w434, w432) -> (w428:errorcluster)
            n175 = Generate User Event(user event=w438, event data cluster="Clear object tab" ("event data"), error in=w428) -> (error out=w439:errorcluster)  [unwired: 1 in, 1 out]
          }
          frame "Update attributes" {
            n176 = property on="Inheritance" class="LstBox (strict)"(error in=w458) -> (error out=w457:errorcluster, "Item Names"=w453:string[])  [unwired: 1 in, 1 out]
            n177 = Not(x="Attributes") -> (.not. x?=w452:bool)
            n178 = Empty String/Path?(string/path="ObjectTree") -> (empty?=w455:bool)
            n179 = Empty Array?(array=w453) -> (empty?=w456:bool)
            n180 = Or(x=w455, y=w456) -> (x .or. y?=w454:bool)
            n181 = case shown="False" w454 {
              tunnel: w457 -> [w497 w587]
              tunnel: w466 -> [_ _]
              tunnel: w465 -> [w496 w585]
              tunnel: "ObjectTree" -> [w478 _]
              tunnel: w452 -> [w477 _]
              tunnel: "Inheritance" -> [w473 _]
              tunnel: [w495 w581] -> w462
              tunnel: w464 -> [w494 w580]
              tunnel: w461 -> [w493 _]
              tunnel: w460 -> [w492 _]
              tunnel: w459 -> [w491 _]
              tunnel: w453 -> [w474 _]
              frame False {
                n182 = Index Array(array=w474, index=w473) -> (element=w472:string)
                n183 = invoke class="Tree (strict)" method="Navigate Tree.Get Parent"(reference=w492, error in=w497, "tag"=w478) -> (error out=w485:errorcluster, "Navigate Tree:Get Parent"=w487:string)  [unwired: 1 in, 2 out]
                n184 = Bundle("ObjectTree"=w478, w477, "Inheritance"=w473) -> (w476:T12)  [unwired: 1 in]
                n185 = Unbundle By Name(w491) -> ("ParPaths"=w490:path[], "ClsPaths"=w486:path[], "ClsNames"=w489:string[])
                n186 = feedback-in #4(w476) -> ()
                n187 = feedback #4(T8 {"ObjectTree"="", "Attributes"=FALSE, "Inheritance"=0}) -> (w481:T8)
                n188 = Equal?(x=w481, y=w476) -> (x = y?=w471:bool)
                n189 = Search 1D Array(1D array=w489, element=w478) -> (index of element=w488:i32)  [unwired: 1 in]
                n190 = Match Pattern(string=w472, regular expression="G#Object" ("string")) -> (offset past match=w480:i32)  [unwired: 1 in, 3 out]
                n191 = Greater Or Equal To 0?(x=w488) -> (x >= 0?=w482:bool)
                n192 = Greater Or Equal To 0?(x=w480) -> (x >= 0?=w470:bool)
                n193 = Select(t=w478, s=w482, f=w487) -> (s? t:f=w483:string)
                n194 = Or(x=w471, y=w470) -> (x .or. y?=w479:bool)
                n195 = case shown="False" w479 {
                  tunnel: w496 -> [_ w521]
                  tunnel: w490 -> [_ w539]
                  tunnel: w489 -> [_ w537]
                  tunnel: w486 -> [_ w536]
                  tunnel: w473 -> [_ w514]
                  tunnel: w493 -> [w499 w531]
                  tunnel: w485 -> [w501 w511]
                  tunnel: [w500 w512] -> w495
                  tunnel: w483 -> [_ w529]
                  tunnel: w477 -> [_ w527]
                  tunnel: w494 -> [w502 w516]
                  tunnel: w470 -> [w498 _]
                  frame True {
                    n196 = case shown="True" w498 {
                      tunnel: w502 -> [_ _]
                      tunnel: w501 -> [w503 w505]
                      tunnel: [w503 w507] -> w500
                      tunnel: w499 -> [_ w506]
                      frame False {
                      }
                      frame True {
                        # "Root class"
                        n197 = invoke on="Invoke Node" class="SubPnl" method="Remove VI"(reference=w506, error in=w505) -> (error out=w504:errorcluster)  [unwired: 1 in, 2 out]
                        n198 = property on="Attributes" class="SubPnl"(error in=w504, "DisabledEnum"=T6."Disabled and Grayed Out" ("Disabled")) -> (error out=w507:errorcluster)  [unwired: 1 in, 1 out]
                      }
                    }
                  }
                  frame False {
                    n199 = in-place {
                      in-place-border: [w540] -> w520
                      n200 = in-place-dvr #5(w521) -> (w541:T4)  [unwired: 1 out]
                      n201 = Unbundle By Name(w541) -> ("vi reference"=w540:refnum<vi>)
                      n202 = in-place-dvr #5(w541) -> (w509:errorcluster)  [unwired: 1 out]
                    }
                    n203 = for {
                      tunnel: w539 -> [w547] mode=indexing
                      tunnel: [w546] -> w538 mode=indexing
                      n204 = Strip Path(path=w547) -> (name=w546:string)  [unwired: 1 out]
                    }
                    n205 = while {
                      tunnel: w537 -> [w561]
                      tunnel: w539 -> [_]
                      tunnel: w538 -> [w557]
                      shift-right: [w558] -> w534
                      shift-left: path[] [] ("ParPaths") -> [w560]
                      shift-right: [w553] -> _
                      shift-left: w529 -> [w559]
                      tunnel: w536 -> [w551]
                      stop <- w548 stop-if-true
                      n206 = Search 1D Array(1D array=w561, element=w559) -> (index of element=w550:i32)  [unwired: 1 in]
                      n207 = Index Array(array=w551, index=w550) -> (element=w549:path)
                      n208 = Index Array(array=w557, index=w550) -> (element=w554:string)
                      n209 = Less Than 0?(x=w550) -> (x < 0?=w552:bool)
                      n210 = Match Pattern(string=w554, regular expression=".lvclass") -> (before substring=w553:string)  [unwired: 1 in, 3 out]
                      n211 = Empty String/Path?(string/path=w553) -> (empty?=w556:bool)
                      n212 = Or(x=w556, y=w552) -> (x .or. y?=w548:bool)
                      n213 = case shown="False" w548 {
                        tunnel: w560 -> [w564 w565]
                        tunnel: [w563 w565] -> w558
                        tunnel: w549 -> [w562 _]
                        frame False {
                          n214 = Build Array (concatenate)(w562, w564) -> (w563:path[])
                        }
                        frame True {
                        }
                      }
                    }
                    n215 = Merge Errors(w511, w509) -> (w510:errorcluster)
                    n216 = Not A Number/Path/Refnum?(number/path/refnum=w520) -> (NaN/Path/Refnum?=w522:bool)
                    n217 = case shown="False" w522 {
                      tunnel: w510 -> [w544 w545]
                      tunnel: w520 -> [w543 _]
                      tunnel: [w542 w545] -> w519
                      frame False {
                        n218 = Close Reference(reference=w543, error in (no error)=w544) -> (error out=w542:errorcluster)
                      }
                      frame True {
                      }
                    }
                    n219 = for {
                      tunnel: w534 -> [w571] mode=indexing
                      tunnel: [w576] -> w528 mode=indexing
                      tunnel: [w575] -> w524 mode=indexing
                      n220 = Strip Path(path=w571) -> (stripped path=w574:path)  [unwired: 1 out]
                      n221 = Build Path(base path=w574, name or relative path="protected") -> (appended path=w573:path)
                      n222 = Build Path(base path=w573, name or relative path="ClassAttributes.ctl") -> (appended path=w576:path)
                      n223 = Build Path(base path=w573, name or relative path="ObjectAttributes.ctl") -> (appended path=w575:path)
                    }
                    n224 = Decrement(x=w514) -> (x-1=w513:i32)
                    n225 = Select(t=w524, s=w527, f=w528) -> (s? t:f=w525:path[])
                    n226 = Index Array(array=w525, index=w513) -> (element=w533:path)
                    n227 = Not(x=w527) -> (.not. x?=w526:bool)
                    n228 = call <vilib>:"G#Debugger_OpenAttributeReference.vi"("vi path"=w533, "error in (no error)"=w519) -> ("vi reference"=w532:refnum<vi>, "error out"=w530:errorcluster)  [unwired: 16 in]
                    n229 = in-place {
                      in-place-border: w528 -> [w569]
                      in-place-border: w524 -> [w568]
                      in-place-border: w532 -> [w566]
                      n230 = in-place-dvr #6(w521) -> (w567:T4)  [unwired: 1 out]
                      n231 = Bundle By Name(cluster=w567, "class attributes"=w569, "object attributes"=w568, "vi reference"=w566) -> (w570:T4)
                      n232 = in-place-dvr #6(w570) -> (w523:errorcluster)  [unwired: 1 out]
                    }
                    n233 = call <vilib>:"G#Debugger_ShowAttributes.vi"("VIRef"=w532, "SubPanel"=w531, "ClassAttributes"=w526, "error in (no error)"=w530) -> ("error out"=w518:errorcluster)  [unwired: 14 in, 1 out]
                    n234 = Generate User Event(user event=w516, event data cluster="UpdateAttrData" ("name or relative path"), error in=w518) -> (error out=w517:errorcluster)  [unwired: 1 in, 1 out]
                    n235 = Merge Errors(w517, w523) -> (w512:errorcluster)
                  }
                }
              }
              frame True {
                # "No item selected in tree"
                n236 = invoke on="Attributes" class="SubPanel" method="Remove VI"(error in=w587) -> (error out=w586:errorcluster)  [unwired: 2 in, 2 out]
                n237 = in-place {
                  in-place-border: w586 -> [w592]
                  in-place-border: [w590] -> w583
                  # "Force a subpanel update!"
                  n238 = in-place-dvr #7(w585) -> (w591:T4)  [unwired: 1 out]
                  n239 = Unbundle By Name(w591) -> ("vi reference"=w588:refnum<vi>)
                  n240 = Not A Number/Path/Refnum?(number/path/refnum=w588) -> (NaN/Path/Refnum?=w589:bool)
                  n241 = case shown="False" w589 {
                    tunnel: w592 -> [w595 w596]
                    tunnel: [w594 w596] -> w590
                    tunnel: w588 -> [w593 _]
                    frame False {
                      n242 = Close Reference(reference=w593, error in (no error)=w595) -> (error out=w594:errorcluster)
                    }
                    frame True {
                    }
                  }
                  n243 = in-place-dvr #7(w591) -> (w584:errorcluster)  [unwired: 1 out]
                }
                n244 = Merge Errors(w584, w583) -> (w582:errorcluster)
                n245 = Generate User Event(user event=w580, event data cluster="Clear object tab" ("event data"), error in=w582) -> (error out=w581:errorcluster)  [unwired: 1 in, 1 out]
              }
            }
            n246 = call <vilib>:"Clear Errors.vi"("error in (no error)"=w462) -> ("error out"=w463:errorcluster)  [unwired: 5 in, 1 out]
          }
          frame "UpdateAttrData" {
            n247 = property class="Tree (strict)"(reference=w610, error in=w609) -> (error out=w601:errorcluster, "Value"=w611:string)  [unwired: 1 out]
            n248 = Unbundle By Name(w612) -> ("Path"=w605:path, "ClsNames"=w608:string[])
            n249 = property on="Inheritance" class="LstBox (strict)"(error in=w601) -> (error out=w600:errorcluster, "Value"=w599:i32)  [unwired: 1 in, 1 out]
            n250 = Search 1D Array(1D array=w608, element=w611) -> (index of element=w607:i32)  [unwired: 1 in]
            n251 = property on="Attributes" class="Bool (strict)"(error in=w600) -> (error out=w603:errorcluster, "Value"=w602:bool)  [unwired: 1 in, 1 out]
            n252 = Not(x=w602) -> (.not. x?=w597:bool)
            n253 = case shown="-1" w607 {
              tunnel: w611 -> [_ w644]
              tunnel: w603 -> [w614 w640]
              tunnel: [w613 w621] -> w606
              tunnel: w605 -> [_ w643]
              tunnel: w604 -> [_ w642]
              tunnel: w597 -> [_ w623]
              tunnel: w599 -> [_ w637]
              tunnel: w598 -> [_ w636]
              frame Default {
                n254 = property on="Attributes" class="SubPnl"(error in=w614, "DisabledEnum"=T6."Disabled and Grayed Out" ("Disabled")) -> (error out=w613:errorcluster)  [unwired: 1 in, 1 out]
              }
              frame -1 {
                # "Get ObjectID"
                n255 = Decrement(x=w637) -> (x-1=w626:i32)
                n256 = Decimal String To Number(string=w644, default (0L)=u32 0 ("default (0 I32)")) -> (number=w624:u32)  [unwired: 1 in, 1 out]
                n257 = To Variant(anything=w624) -> (Variant=w639:variant)
                n258 = To Variant(anything=w623) -> (Variant=w638:variant)
                n259 = Build Array(w639, w638) -> (w619:variant[])
                n260 = Select(t="attributes" ("y"), s=w623, f="class attributes" ("y")) -> (s? t:f=w635:string)
                n261 = call <vilib>:"G#Debugger_RunMethod.vi"("ClassPath"=w643, "MethodName"="GetAttributeValue.vi" ("name or relative path"), "ClassPrefix"=w642, "error in (no error)"=w640, "ControlValue"=w619) -> ("ControlValue out"=w631:variant[], "error out"=w618:errorcluster)  [unwired: 12 in, 1 out]
                n262 = Index Array(array=w631, index=w626) -> (element=w628:variant)
                n263 = in-place {
                  in-place-border: [w652] -> w632
                  n264 = in-place-dvr #8(w636) -> (w653:T4)  [unwired: 1 out]
                  n265 = Unbundle By Name(w653) -> ("vi reference"=w652:refnum<vi>)
                  n266 = in-place-dvr #8(w653) -> (w616:errorcluster)  [unwired: 1 out]
                }
                n267 = Merge Errors(w618, w616) -> (w617:errorcluster)
                n268 = invoke class="VI" method="Ctrl Val.Get"(reference=w632, error in=w617, "Control Name"=w635) -> (reference out=w627:refnum<vi>, error out=w633:errorcluster, "Get Control Value Variant"=w634:variant)  [unwired: 1 in, 1 out]
                n269 = Not Equal?(x=w634, y=w628) -> (x != y?=w625:bool)
                n270 = case shown="True" w625 {
                  tunnel: [w646 w647] -> w620
                  tunnel: w633 -> [w646 w651]
                  tunnel: w627 -> [_ w650]
                  tunnel: w635 -> [_ w649]
                  tunnel: w628 -> [_ w648]
                  frame False {
                  }
                  frame True {
                    n271 = invoke class="VI" method="Ctrl Val.Set"(reference=w650, error in=w651, "Control Name"=w649, "Value"=w648) -> (error out=w647:errorcluster)  [unwired: 1 in, 4 out]
                  }
                }
                n272 = property on="Attributes" class="SubPnl"(error in=w620, "DisabledEnum"=T6."Enabled" ("Disabled")) -> (error out=w621:errorcluster)  [unwired: 1 in, 1 out]
              }
            }
          }
          frame "Run VI" {
            n273 = disable-structure shown="Enabled" {
              disable-tunnel: w656 -> [w663 w702]
              disable-tunnel: [w662 w702] -> w655
              frame Disabled {
                n274 = property on="DebugTree" class="Tree (strict)"() -> ("Value"=w657:string)  [unwired: 2 in, 2 out]
                n275 = Match Pattern(string=w657, regular expression="[.][v][i]") -> (before substring=w660:string, match substring=w659:string)  [unwired: 1 in, 2 out]
                n276 = Concatenate Strings(w660, w659) -> (w658:string)
                n277 = String To Path(string=w658) -> (path=w664:path)
                n278 = Open VI Reference(vi path=w664, error in (no error)=w663) -> (vi reference=w666:refnum<vi>, error out=w665:errorcluster)  [unwired: 4 in]
                n279 = case shown="No Error" w665 {
                  selector: w665 -> [w671 _]
                  tunnel: [w677 errorcluster {"status"=FALSE, "code"=0, "source"=""} ("error in (no error)")] -> w662
                  tunnel: w666 -> [w670 _]
                  tunnel: w664 -> [w675 _]
                  frame No Error {
                    n280 = stacked-sequence {
                      tunnel: w675 -> [w683]
                      tunnel: [w683] -> w674
                      frame #0 {
                        "Run State" <- "Running..." ("Run State")
                      }
                    }
                    n281 = property class="VI"(reference=w670, error in=w671) -> (error out=w668:errorcluster, "Exec.State"=w669:T13, "Exec.IsReentrant"=w672:bool)  [unwired: 1 out]
                    n282 = case shown="\"Run top level\"" w669 {
                      tunnel: [FALSE TRUE w680 w681] -> w673
                      tunnel: w672 -> [_ _ w680 w681]
                      frame Default {
                      }
                      frame "Idle" {
                      }
                      frame "Run top level" {
                      }
                      frame "Running" {
                      }
                    }
                    n283 = case shown="True" w673 {
                      tunnel: [w689 w697] -> w676
                      tunnel: w668 -> [w689 w692]
                      tunnel: w674 -> [w688 _]
                      tunnel: [w685 w700] -> w667
                      tunnel: w669 -> [w684 _]
                      tunnel: w670 -> [_ w693]
                      frame False {
                        n284 = Strip Path(path=w688) -> (name=w687:string)  [unwired: 1 out]
                        n285 = Format Into String(format string="%s is not reentrant or in idle execution state! (%s)", w687, w684) -> (resulting string=w685:string)  [unwired: 2 in, 1 out]
                      }
                      frame True {
                        n286 = call <vilib>:"G#Debugger_RunVI.vi"("vi reference"=w693, "wait until done"="Wait Until Done", "error in (no error)"=w692) -> ("class name"=→"Cached Reference Class Name":string, "object ID"=→"CachedObjId":u32, "message"=w696:string, "not a refnum?"=w691:bool, "error out"=w697:errorcluster)  [unwired: 12 in]
                        n287 = Not(x=w691) -> (.not. x?=→"Cached Ref Valid":bool)
                        n288 = Select(t=w696, s="Wait Until Done", f="Run state is not available!") -> (s? t:f=w700:string)
                      }
                    }
                    n289 = property on="Run State" class="Str"("Value"=w667) -> ()  [unwired: 2 in, 2 out]
                    n290 = Close Reference(reference=w670, error in (no error)=w676) -> (error out=w677:errorcluster)
                  }
                  frame Error {
                  }
                }
              }
              frame Enabled {
              }
            }
          }
          frame "Wait".."Wb" {
            n291 = Decimal String To Number(string=w708, offset=5, default (0L)=u32 0 ("default (0 I32)")) -> (number=w705:u32)  [unwired: 1 out]
            n292 = Wait (ms)(milliseconds to wait=w705) -> ()  [unwired: 1 out]
          }
          frame "Highlight aggregates" {
            n293 = property on="Property Node" class="Tree (strict)"(reference=w711, error in=w716) -> (error out=w715:errorcluster, "Value"=w713:string)  [unwired: 1 out]
            n294 = disable-structure shown="Disabled" {
              disable-tunnel: w715 -> [w726 w760]
              disable-tunnel: w714 -> [w725 _]
              disable-tunnel: w713 -> [w724 _]
              disable-tunnel: [w722 w760] -> w712
              disable-tunnel: w711 -> [w721 _]
              disable-tunnel: w710 -> [w717 _]
              frame Disabled {
                n295 = call <vilib>:"G#Debugger_GetObjectFromTag.vi"("Objects dvr"=w725, "Tag"=w724, "class attributes"=FALSE, "error in (no error)"=w726) -> ("Ref"=w720:refnum<class "G#Object.lvclass">, "Found"=w718:bool, "error out"=w719:errorcluster)  [unwired: 13 in]
                n296 = case shown="True" w718 {
                  tunnel: [w727 w735] -> w722
                  tunnel: w721 -> [_ w747]
                  tunnel: w720 -> [_ w746]
                  tunnel: w719 -> [w727 w744]
                  tunnel: w717 -> [_ w734]
                  frame False {
                  }
                  frame True {
                    w741 = TRUE  # remove duplicates
                    # "redraw FP"
                    n297 = property on="Attributes" class="Bool (strict)"(error in=w744) -> (error out=w743:errorcluster, "Value"=w742:bool)  [unwired: 1 in, 1 out]
                    n298 = call <vilib>:"G#Object_GetAggregatedObjects.vi"("reference in"=w746, "class attributes (F)"=w742, "remove duplicates (F)"=w741, "error in (no error)"=w743) -> ("aggregated objects"=w740:refnum<class "G#Object.lvclass">[], "error out"=w739:errorcluster)  [unwired: 12 in, 2 out]
                    n299 = for {
                      tunnel: w740 -> [w750] mode=indexing
                      shift-right: [w751] -> w745
                      shift-left: w739 -> [w753]
                      tunnel: [w752] -> w728 mode=indexing if=w748
                      n300 = call-dynamic "NotARefNum.vi"("reference in"=w750) -> ("not a refnum?"=w749:bool)  [unwired: 1 in, 1 out]
                      n301 = case shown="False" w749 {
                        tunnel: w750 -> [w758 _]
                        tunnel: w753 -> [w757 w759]
                        tunnel: [w755 _] -> w752
                        tunnel: [w754 w759] -> w751
                        frame False {
                          # "ObjectIDs are the\ntags in the object tree"
                          n302 = call-dynamic "GetObjectID.vi"("reference in"=w758, "error in (no error)"=w757) -> ("object ID"=w756:u32, "error out"=w754:errorcluster)  [unwired: 15 in, 1 out]
                          n303 = Number To Decimal String(number=w756) -> (decimal integer string=w755:string)  [unwired: 1 in]
                        }
                        frame True {
                        }
                      }
                      n304 = Not(x=w749) -> (.not. x?=w748:bool)
                    }
                    n305 = control-ref of="Aggregates"() -> (w733:refnum<vi>)
                    n306 = control-ref of="AggregatesTags"() -> (w732:refnum<vi>)
                    n307 = Array Size(array=w728) -> (size(s)=w731:i32)
                    n308 = call <vilib>:"G#Debugger_Highlight.vi"("Tree"=w747, "Aggregates"=w733, "ObjectIDs"=w728, "error in (no error)"=w745, "AggregatesTags"=w732) -> ("error out"=w736:errorcluster)  [unwired: 14 in]
                    n309 = Greater Or Equal?(x=w731, y=8) -> (x >= y?=w730:bool)
                    n310 = property class="Pnl"(reference=w734, error in=w736, "DeferPanUpdts"=FALSE ("Defer Panel Updates"), "DeferPanUpdts"=TRUE ("Defer Panel Updates")) -> (error out=w735:errorcluster)  [unwired: 1 out]
                    n311 = property on="Aggregates" class="LstBox (strict)"("Scrollbar Visible"=w730) -> ()  [unwired: 2 in, 2 out]
                  }
                }
              }
              frame Enabled {
              }
            }
          }
          frame "ListAggregators" {
            n312 = property on="Property Node" class="Tree (strict)"(reference=w763, error in=w768) -> (error out=w767:errorcluster, "Value"=w765:string)  [unwired: 1 out]
            n313 = disable-structure shown="Disabled" {
              disable-tunnel: w767 -> [w778 w874]
              disable-tunnel: w766 -> [w777 _]
              disable-tunnel: w765 -> [w776 _]
              disable-tunnel: [w774 w874] -> w764
              disable-tunnel: w763 -> [w773 _]
              disable-tunnel: w762 -> [w769 _]
              frame Disabled {
                n314 = call <vilib>:"G#Debugger_GetObjectFromTag.vi"("Objects dvr"=w777, "Tag"=w776, "class attributes"=FALSE, "error in (no error)"=w778) -> ("Ref"=w772:refnum<class "G#Object.lvclass">, "Found"=w770:bool, "error out"=w771:errorcluster)  [unwired: 13 in]
                n315 = case shown="True" w770 {
                  tunnel: [w779 w799] -> w774
                  tunnel: w773 -> [_ _]
                  tunnel: w772 -> [_ w798]
                  tunnel: w771 -> [w779 w804]
                  tunnel: w769 -> [_ w784]
                  frame False {
                  }
                  frame True {
                    # "redraw FP"
                    n316 = call-dynamic "GetObjectID.vi"("reference in"=w798) -> ("object ID"=w781:u32)  [unwired: 16 in, 2 out]
                    n317 = property on="Attributes" class="Bool (strict)"(error in=w804) -> (error out=w803:errorcluster, "Value"=w802:bool)  [unwired: 1 in, 1 out]
                    n318 = Equal To 0?(x=w781) -> (x = 0?=w780:bool)
                    n319 = case shown="False" w780 {
                      tunnel: w803 -> [w816 w867]
                      tunnel: w802 -> [w815 _]
                      tunnel: w781 -> [w809 _]
                      tunnel: [w808 w867] -> w797
                      tunnel: [w806 _] -> w790
                      tunnel: [w805 _] -> w788
                      frame False {
                        w814 = TRUE  # remove duplicates
                        n320 = call <vilib>:"G#Object_GetAllObjects.vi"("only refs (F)"=TRUE) -> ("all refs"=w811:refnum<class "G#Object.lvclass">[])  [unwired: 15 in, 3 out]
                        n321 = for {
                          tunnel: w815 -> [w823]
                          tunnel: w814 -> [w822]
                          tunnel: [w820] -> w813 mode=indexing if=w817
                          shift-right: [w821] -> w812
                          shift-left: w816 -> [w824]
                          tunnel: w811 -> [w819] mode=indexing
                          tunnel: [w819] -> w807 mode=indexing if=w817
                          n322 = call-dynamic "NotARefNum.vi"("reference in"=w819) -> ("not a refnum?"=w818:bool)  [unwired: 1 in, 1 out]
                          n323 = Not(x=w818) -> (.not. x?=w817:bool)
                          n324 = case shown="False" w818 {
                            tunnel: w824 -> [w831 w836]
                            tunnel: w823 -> [w830 _]
                            tunnel: w822 -> [w829 _]
                            tunnel: [w828 w836] -> w821
                            tunnel: w819 -> [w827 _]
                            tunnel: [w825 _] -> w820
                            frame False {
                              n325 = call <vilib>:"G#Object_GetAggregatedObjects.vi"("reference in"=w827, "class attributes (F)"=w830, "remove duplicates (F)"=w829, "error in (no error)"=w831) -> ("aggregated objects"=w826:refnum<class "G#Object.lvclass">[], "error out"=w828:errorcluster)  [unwired: 12 in, 2 out]
                              n326 = for {
                                tunnel: w826 -> [w835] mode=indexing
                                tunnel: [w834] -> w825 mode=indexing if=w832
                                n327 = call-dynamic "NotARefNum.vi"("reference in"=w835) -> ("not a refnum?"=w833:bool, "reference out"=w834:refnum<class "G#Object.lvclass">)  [unwired: 1 in]
                                n328 = Not(x=w833) -> (.not. x?=w832:bool)
                              }
                            }
                            frame True {
                            }
                          }
                        }
                        n329 = for {
                          tunnel: w813 -> [w847] mode=indexing
                          shift-right: [w843] -> w808
                          shift-left: w812 -> [w846]
                          tunnel: [w839] -> w806 mode=indexing if=w837
                          tunnel: w809 -> [w845]
                          tunnel: w807 -> [w842] mode=indexing
                          tunnel: [w838] -> w805 mode=indexing if=w837
                          # "ObjectIDs are the\ntags in the object tree"
                          n330 = for {
                            tunnel: w847 -> [w858] mode=indexing
                            tunnel: w845 -> [w856]
                            tunnel: [w853] -> w837
                            shift-right: [w854] -> w844
                            shift-left: w846 -> [w857]
                            stop <- w853 stop-if-true
                            n331 = call-dynamic "GetObjectID.vi"("reference in"=w858, "error in (no error)"=w857) -> ("object ID"=w855:u32, "error out"=w854:errorcluster)  [unwired: 15 in, 1 out]
                            n332 = Equal?(x=w856, y=w855) -> (x = y?=w853:bool)
                          }
                          n333 = case shown="True" w837 {
                            tunnel: w844 -> [w859 w866]
                            tunnel: [w859 w865] -> w843
                            tunnel: w842 -> [_ w861]
                            tunnel: [_ w863] -> w841
                            tunnel: [_ w862] -> w840
                            tunnel: [_ w860] -> w838
                            frame False {
                            }
                            frame True {
                              n334 = call-dynamic "GetObjectID.vi"("reference in"=w861) -> ("object ID"=w860:u32)  [unwired: 16 in, 2 out]
                              n335 = call-dynamic "GetObjectStatus.vi"("reference in"=w861, "simple info (F)"=TRUE, "error in (no error)"=w866) -> ("class name"=w863:string, "object name"=w862:string, "error out"=w865:errorcluster)  [unwired: 5 in, 9 out]
                            }
                          }
                          n336 = disable-structure shown="Enabled" {
                            disable-tunnel: w841 -> [w851 _]
                            disable-tunnel: w840 -> [w850 w852]
                            disable-tunnel: [w848 w852] -> w839
                            frame Enabled {
                              n337 = Format Into String(format string="%s:%s", w851, w850) -> (resulting string=w848:string)  [unwired: 2 in, 1 out]
                            }
                            frame Disabled {
                            }
                          }
                        }
                      }
                      frame True {
                      }
                    }
                    n338 = for {
                      tunnel: w788 -> [w872] mode=indexing
                      tunnel: w790 -> [w873] mode=indexing
                      tunnel: [w871] -> w792 mode=indexing
                      n339 = Bundle(cluster=T9 {"Active Item Row Number"=0, "name"=""}, "Active Item Row Number"=w872, "name"=w873) -> (w871:T9)
                    }
                    n340 = Sort 1D Array(array=w788) -> (sorted array=w787:u32[])
                    n341 = Array Size(array=w787) -> (size(s)=w795:i32)
                    n342 = Greater Or Equal?(x=w795, y=7) -> (x >= y?=w794:bool)
                    n343 = Number To Decimal String(number=w787) -> (decimal integer string=w785:string[])  [unwired: 1 in]
                    n344 = property on="Aggregators" class="LstBox (strict)"("Scrollbar Visible"=w794) -> ()  [unwired: 2 in, 2 out]
                    n345 = Sort 1D Array(array=w792) -> (sorted array=w791:T14)
                    n346 = for {
                      tunnel: w791 -> [w869] mode=indexing
                      tunnel: [w868] -> w789 mode=indexing
                      n347 = Unbundle By Name(w869) -> ("name"=w868:string)
                    }
                    n348 = property on="Aggregators" class="LstBox (strict)"(error in=w797, "Item Names"=w789) -> (error out=w796:errorcluster)  [unwired: 1 in, 1 out]
                    n349 = control-ref of="AggregatorsTags"() -> (w793:refnum<vi>)
                    n350 = property on="Property Node" class="LstBox (strict)"(reference=w793, "Item Names"=w785, "Value"=-1, "Top Row"=0) -> ()  [unwired: 1 in, 2 out]
                    n351 = property class="Pnl"(reference=w784, error in=w796, "DeferPanUpdts"=FALSE ("Defer Panel Updates"), "DeferPanUpdts"=TRUE ("Defer Panel Updates")) -> (error out=w799:errorcluster)  [unwired: 1 out]
                  }
                }
              }
              frame Enabled {
              }
            }
          }
          frame "Connected", "Disconnected" {
            n352 = Equal?(x=w878, y="Connected") -> (x = y?=→"Connected?":bool)
          }
        }
        n353 = call <vilib>:"Unset Busy.vi"("error in (no error)"=w156) -> ("error out"=w155:errorcluster)  [unwired: 10 in]
      }
      event User Event {
        n354 = event-data() -> ("GUI event"=w884:string)  [unwired: 1 in]
        n355 = case shown="\"Exit\"" w884 {
          tunnel: w883 -> [w885 w887]
          tunnel: [w885 w886] -> w882
          tunnel: w881 -> [_ w890]
          frame Default {
          }
          frame "Exit" {
            n356 = Unbundle By Name(w890) -> ("CloneUIevent"=w889:refnum<user-event>)
            n357 = Generate User Event(user event=w889, event data cluster="Exit" ("event data"), error in=w887) -> (error out=w886:errorcluster)  [unwired: 1 in, 1 out]
          }
        }
      }
      event "Aggregates": Double Click {
        n358 = event-data() -> ()  [unwired: 1 in, 1 out]
        n359 = control-ref of="AggregatesTags"() -> (w893:refnum<vi>)
        n360 = control-ref of="Aggregates"() -> (w892:refnum<vi>)
        n361 = property class="LstBox (strict)"(reference=w893) -> ("Item Names"=w897:string[])  [unwired: 1 in, 2 out]
        n362 = property class="LstBox (strict)"(reference=w892) -> ("Value"=w898:i32)  [unwired: 1 in, 2 out]
        n363 = Index Array(array=w897, index=w898) -> (element=w896:string)
        n364 = property class="Tree (strict)"(reference=w895, "Val(Sgnl)"=w896) -> ()  [unwired: 1 in, 2 out]
      }
      event "Aggregators": Double Click {
        n365 = event-data() -> ()  [unwired: 1 in, 1 out]
        n366 = control-ref of="Aggregators"() -> (w900:refnum<vi>)
        n367 = control-ref of="AggregatorsTags"() -> (w901:refnum<vi>)
        n368 = property class="LstBox (strict)"(reference=w900) -> ("Value"=w906:i32)  [unwired: 1 in, 2 out]
        n369 = property class="LstBox (strict)"(reference=w901) -> ("Item Names"=w905:string[])  [unwired: 1 in, 2 out]
        n370 = Index Array(array=w905, index=w906) -> (element=w904:string)
        n371 = property class="Tree (strict)"(reference=w903, "Val(Sgnl)"=w904) -> ()  [unwired: 1 in, 2 out]
      }
      event "ShowAggregators": Value Change {
        n372 = event-data() -> ("NewVal"=w909:bool)  [unwired: 1 in]
        n373 = Unbundle By Name(w911) -> ("CloneUIevent"=w910:refnum<user-event>)
        n374 = property on="Aggregators" class="LstBox (strict)"("Visible"=w909) -> ()  [unwired: 2 in, 2 out]
        n375 = case shown="True" w909 {
          tunnel: w913 -> [w915 w919]
          tunnel: [w915 w918] -> w912
          tunnel: w910 -> [_ w917]
          tunnel: [u32 16 ("Number of Rows") u32 7 ("Number of Rows")] -> w908
          frame False {
          }
          frame True {
            n376 = Generate User Event(user event=w917, event data cluster="ListAggregators" ("event data"), error in=w919) -> (error out=w918:errorcluster)  [unwired: 1 in, 1 out]
          }
        }
        n377 = property on="Aggregates" class="LstBox (strict)"("Number of Rows"=w908) -> ()  [unwired: 2 in, 2 out]
      }
      event Panel Close? {
        n378 = event-data() -> ()  [unwired: 1 in, 3 out]
        n379 = Unbundle By Name(w926) -> ("CloneUIevent"=w923:refnum<user-event>)
        n380 = Generate User Event(user event=w923, event data cluster="Exit" ("event data"), error in=w928) -> (error out=w927:errorcluster)  [unwired: 1 in, 1 out]
        n381 = event-data("Discard?"=TRUE) -> ()  [unwired: 1 in, 1 out]
      }
      event "Tab Control": Value Change {
        n382 = event-data() -> ("NewVal"=w934:enum32{"Objects", "Trace", "Active Debug"})  [unwired: 1 in]
        n383 = Unbundle By Name(w931) -> ("CloneUIevent"=w930:refnum<user-event>)
        n384 = case shown="\"Objects\"" w934 {
          tunnel: w933 -> [w938 w941]
          tunnel: [w940 w941] -> w932
          tunnel: w930 -> [w936 _]
          frame "Objects" {
            # "Refresh tree control"
            n385 = Generate User Event(user event=w936, event data cluster="Clear object tab" ("event data"), error in=w938) -> (error out=w937:errorcluster)  [unwired: 1 in, 1 out]
            n386 = Generate User Event(user event=w936, event data cluster="Refresh" ("event data"), error in=w937) -> (error out=w940:errorcluster)  [unwired: 1 in, 1 out]
          }
          frame Default {
          }
        }
      }
      event "ObjectTree": Value Change {
        n387 = event-data() -> ()  [unwired: 1 in, 1 out]
        n388 = property class="Tree (strict)"(reference=w985, error in=w986) -> (reference out=w958:refnum<vi>, error out=w962:errorcluster, "Value"=w956:string)
        n389 = Unbundle By Name(w983) -> ("ClassInfoDvr"=w957:refnum<data-value>, "CloneUIevent"=w979:refnum<user-event>)
        n390 = Unbundle By Name(w969) -> ("ParPaths"=w968:path[], "ClsNames"=w964:string[])
        n391 = Search 1D Array(1D array=w964, element=w956) -> (index of element=w963:i32)  [unwired: 1 in]
        n392 = invoke class="Tree (strict)" method="Navigate Tree.Get Parent"(reference=w958, error in=w962, "tag"=w956) -> (error out=w944:errorcluster, "Navigate Tree:Get Parent"=w961:string)  [unwired: 1 in, 2 out]
        n393 = Greater Or Equal To 0?(x=w963) -> (x >= 0?=w960:bool)
        n394 = Select(t="", s=w960, f=w956) -> (s? t:f=w955:string)
        n395 = Decimal String To Number(string=w955, default (0L)=u32 0 ("default (0 I32)")) -> (number=w953:u32)  [unwired: 1 in, 1 out]
        "Object ID" <- w953
        n396 = Select(t=w956, s=w960, f=w961) -> (s? t:f=w947:string)
        n397 = in-place {
          in-place-border: [w1001] -> w948
          n398 = in-place-dvr #9(w957) -> (w1001:T1)  [unwired: 1 out]
          n399 = in-place-dvr #9(w1001) -> (w943:errorcluster)  [unwired: 1 out]
        }
        n400 = Merge Errors(w944, w943) -> (w942:errorcluster)
        n401 = for {
          tunnel: w948 -> [w995] mode=indexing
          tunnel: [w994] -> w946
          tunnel: w947 -> [w993]
          tunnel: [w990] -> w945
          stop <- w991 stop-if-true
          n402 = Unbundle By Name(w995) -> ("ClassName"=w992:string, "Owner"=w994:string, "FullClassName"=w990:string)
          n403 = Equal?(x=w993, y=w992) -> (x = y?=w991:bool)
        }
        "Full Class Name" <- w945
        "Owner" <- w946
        n404 = for {
          tunnel: w948 -> [w1000] mode=indexing
          tunnel: [w999] -> w951
          tunnel: w953 -> [w998]
          tunnel: [w996] -> w952
          stop <- w996 stop-if-true
          n405 = Unbundle By Name(w1000) -> ("ObjectID"=w997:u32, "ObjectName"=w999:string)
          n406 = Equal?(x=w998, y=w997) -> (x = y?=w996:bool)
        }
        n407 = Build Array(w947) -> (w966:string[])
        n408 = property on="CachedObjId" class="DigNum (strict)"("Value"=w953) -> ()  [unwired: 2 in, 2 out]
        n409 = for {
          tunnel: w968 -> [w1003] mode=indexing
          tunnel: [w1002] -> w967 mode=indexing
          n410 = Strip Path(path=w1003) -> (name=w1002:string)  [unwired: 1 out]
        }
        n411 = Select(t=w951, s=w952, f="") -> (s? t:f=→"Object Name":string)
        n412 = while {
          tunnel: w964 -> [w1015]
          tunnel: w968 -> [_]
          tunnel: w967 -> [w1011]
          shift-right: [w1012] -> w965
          shift-left: w966 -> [w1014]
          shift-right: [w1004] -> _
          shift-left: w947 -> [w1013]
          stop <- w1007 stop-if-true
          n413 = Search 1D Array(1D array=w1015, element=w1013) -> (index of element=w1010:i32)  [unwired: 1 in]
          n414 = Index Array(array=w1011, index=w1010) -> (element=w1005:string)
          n415 = Match Pattern(string=w1005, regular expression=".lvclass") -> (before substring=w1004:string)  [unwired: 1 in, 3 out]
          n416 = Less Than 0?(x=w1010) -> (x < 0?=w1008:bool)
          n417 = Empty String/Path?(string/path=w1004) -> (empty?=w1009:bool)
          n418 = Or(x=w1009, y=w1008) -> (x .or. y?=w1007:bool)
          n419 = case shown="False" w1007 {
            tunnel: w1014 -> [w1018 w1019]
            tunnel: [w1017 w1019] -> w1012
            tunnel: w1004 -> [w1016 _]
            frame False {
              n420 = Build Array (concatenate)(w1016, w1018) -> (w1017:string[])
            }
            frame True {
            }
          }
        }
        n421 = case shown="True" "Highlight Aggregates?" {
          tunnel: w942 -> [w1025 w1029]
          tunnel: [w1025 w1028] -> w980
          tunnel: w979 -> [_ w1026]
          frame False {
          }
          frame True {
            n422 = Generate User Event(user event=w1026, event data cluster="Highlight aggregates" ("event data"), error in=w1029) -> (error out=w1028:errorcluster)  [unwired: 1 in, 1 out]
          }
        }
        n423 = Array Size(array=w965) -> (size(s)=w971:i32)
        n424 = property on="Cached Reference Class Name" class="Str"("Value"="" ("Cached Reference Class Name")) -> ()  [unwired: 2 in, 2 out]
        n425 = Generate User Event(user event=w979, event data cluster="Update attributes" ("event data"), error in=w980) -> (user event out=w975:refnum<user-event>, error out=w977:errorcluster)  [unwired: 1 in]
        n426 = Decrement(x=w971) -> (x-1=w984:i32)
        n427 = Greater Or Equal?(x=w971, y=8) -> (x >= y?=w973:bool)
        n428 = case shown="True" "ShowAggregators" {
          tunnel: w977 -> [w1020 w1023]
          tunnel: [w1020 w1022] -> w976
          tunnel: w975 -> [_ w1021]
          frame False {
          }
          frame True {
            n429 = Generate User Event(user event=w1021, event data cluster="ListAggregators" ("event data"), error in=w1023) -> (error out=w1022:errorcluster)  [unwired: 1 in, 1 out]
          }
        }
        n430 = property on="Inheritance" class="LstBox (strict)"("Scrollbar Visible"=w973) -> ()  [unwired: 2 in, 2 out]
        n431 = property on="Inheritance" class="LstBox (strict)"("Item Names"=w965, "Value"=w984, "Top Row"=0) -> ()  [unwired: 2 in, 2 out]
        n432 = call <vilib>:"Clear Errors.vi"("error in (no error)"=w976) -> ("error out"=w981:errorcluster)  [unwired: 5 in, 1 out]
        "# of Users" <- 0 ("# of Users")
        "Counter" <- FALSE ("Counter")
      }
      event "DebugTree": Value Change {
        n433 = event-data() -> ("NewVal"=w1035:string)  [unwired: 1 in, 4 out]
        n434 = Match Pattern(string=w1035, regular expression="[.][v][i]") -> (before substring=w1033:string, match substring=w1032:string)  [unwired: 1 in, 2 out]
        n435 = Concatenate Strings(w1033, w1032) -> (w1031:string)
        n436 = String To Path(string=w1031) -> (path=w1036:path)
        n437 = Open VI Reference(vi path=w1036, error in (no error)=w1041) -> (vi reference=w1039:refnum<vi>, error out=w1038:errorcluster)  [unwired: 4 in]
        n438 = case shown="No Error" w1038 {
          selector: w1038 -> [w1045 _]
          tunnel: [w1048 w1058] -> w1040
          tunnel: w1039 -> [w1043 _]
          tunnel: [w1046 w1059] -> w1037
          frame No Error {
            n439 = call <vilib>:"G#Debugger_SetCachedRef.vi"("MethodVIref"=w1043, "error in (no error)"=w1045) -> ("error out"=w1044:errorcluster)  [unwired: 17 in]
            n440 = invoke on="Method VI Panel" class="SubPanel" method="Insert VI"(error in=w1044, "VI Ref"=w1043) -> (error out=w1042:errorcluster)  [unwired: 2 in, 3 out]
            n441 = case shown="No Error" w1042 {
              selector: w1042 -> [w1052 _]
              tunnel: [w1051 w1054] -> w1047
              tunnel: w1043 -> [w1053 _]
              tunnel: [w1049 w1056] -> w1046
              frame No Error {
                n442 = invoke class="VI" method="VI Icon.Get as Image Data"(reference=w1053, error in=w1052) -> (error out=w1051:errorcluster, "ImageData"=w1050:T15)  [unwired: 4 in, 4 out]
                n443 = call <vilib>:"Draw Flattened Pixmap.vi"("image data"=w1050) -> ("new picture"=w1049:picture)  [unwired: 8 in]
              }
              frame Error {
                n444 = vi-ref "G#Debugger.lvlib:G#Debugger_DebugDialog.vi"() -> (w1055:refnum<vi>)
                n445 = invoke on="Method VI Panel" class="SubPanel" method="Insert VI"("VI Ref"=w1055) -> (error out=w1054:errorcluster)  [unwired: 3 in, 3 out]
                n446 = call "Empty Picture"() -> ("empty picture"=w1056:picture)
              }
            }
            n447 = Close Reference(reference=w1043, error in (no error)=w1047) -> (error out=w1048:errorcluster)
          }
          frame Error {
            n448 = invoke on="Method VI Panel" class="SubPanel" method="Remove VI"(error in=errorcluster {"status"=FALSE, "code"=0, "source"=""} ("error in (no error)")) -> (error out=w1058:errorcluster)  [unwired: 2 in, 2 out]
            n449 = call "Empty Picture"() -> ("empty picture"=w1059:picture)
          }
        }
        "Icon" <- w1037
      }
      event "Run VI": Value Change {
        # "We need to fire a new event so we don't lock up the UI event."
        n450 = event-data() -> ()  [unwired: 1 in, 1 out]
        n451 = Unbundle By Name(w1061) -> ("CloneUIevent"=w1064:refnum<user-event>)
        n452 = Generate User Event(user event=w1064, event data cluster="Run VI" ("event data"), error in=w1063) -> (error out=w1062:errorcluster)  [unwired: 1 in, 1 out]
      }
      event "Attributes": Value Change {
        n453 = event-data() -> ()  [unwired: 1 in, 5 out]
        n454 = property class="Tree (strict)"(reference=w1070, error in=w1071) -> (reference out=w1068:refnum<vi>, error out=w1069:errorcluster, "Value"=w1067:string)
        n455 = property class="Tree (strict)"(reference=w1068, error in=w1069, "Val(Sgnl)"=w1067) -> (error out=w1072:errorcluster)  [unwired: 1 out]
      }
      event "Inheritance": Value Change {
        n456 = event-data() -> ()  [unwired: 1 in, 1 out]
        n457 = Unbundle By Name(w1075) -> ("CloneUIevent"=w1077:refnum<user-event>)
        n458 = Generate User Event(user event=w1077, event data cluster="Update attributes" ("event data"), error in=w1076) -> (error out=w1074:errorcluster)  [unwired: 1 in, 1 out]
      }
      event "Refresh", "Hide Empty Classes?": Value Change {
        n459 = event-data() -> ()  [unwired: 1 in, 1 out]
        n460 = Unbundle By Name(w1083) -> ("CloneUIevent"=w1080:refnum<user-event>)
        n461 = Generate User Event(user event=w1080, event data cluster="Refresh" ("event data"), error in=w1084) -> (error out=w1082:errorcluster)  [unwired: 1 in, 1 out]
      }
      event "Clear": Value Change {
        n462 = event-data() -> ()  [unwired: 1 in, 1 out]
        n463 = Unbundle By Name(w1087) -> ("Path"=w1086:path)
        n464 = To Variant(anything="Debugger clearing display!" ("Control Name")) -> (Variant=w1091:variant)
        n465 = Build Array(w1091) -> (w1085:variant[])
        n466 = call <vilib>:"G#Debugger_RunMethod.vi"("ClassPath"=w1086, "MethodName"="SendUserEvent.vi" ("name or relative path"), "ClassPrefix"=w1090, "error in (no error)"=w1089, "ControlValue"=w1085) -> ("error out"=w1088:errorcluster)  [unwired: 12 in, 2 out]
        n467 = property on="Trace" class="Str"(error in=w1088, "Value"="") -> (error out=w1095:errorcluster)  [unwired: 1 in, 1 out]
      }
      event "Garbage collect": Value Change {
        n468 = event-data() -> ()  [unwired: 1 in, 1 out]
        n469 = Unbundle By Name(w1112) -> ("CloneUIevent"=w1111:refnum<user-event>)
        n470 = Unbundle By Name(w1106) -> ("Path"=w1099:path)
        n471 = To Variant(anything="Debugger garbage collected!" ("Control Name")) -> (Variant=w1103:variant)
        n472 = Build Array(w1103) -> (w1096:variant[])
        n473 = call <vilib>:"G#Debugger_RunMethod.vi"("ClassPath"=w1099, "MethodName"="SendUserEvent.vi" ("name or relative path"), "ClassPrefix"=w1098, "error in (no error)"=w1102, "ControlValue"=w1096) -> ("error out"=w1101:errorcluster)  [unwired: 12 in, 2 out]
        n474 = To Variant(anything=FALSE) -> (Variant=w1107:variant)
        n475 = Build Array(w1107) -> (w1097:variant[])
        n476 = call <vilib>:"G#Debugger_RunMethod.vi"("ClassPath"=w1099, "MethodName"="GarbageCollector.vi", "ClassPrefix"=w1098, "error in (no error)"=w1101, "ControlValue"=w1097) -> ("error out"=w1100:errorcluster)  [unwired: 12 in, 2 out]
        n477 = property on="Enable Active Debug" class="Bool (strict)"() -> ("Value"=w1116:bool)  [unwired: 2 in, 2 out]
        n478 = call <vilib>:"Clear Errors.vi"("error in (no error)"=w1100) -> ("error out"=w1110:errorcluster)  [unwired: 5 in, 1 out]
        n479 = case shown="True" w1116 {
          tunnel: w1110 -> [w1117 w1122]
          tunnel: [w1117 w1121] -> w1113
          tunnel: w1099 -> [_ w1120]
          tunnel: w1098 -> [_ w1119]
          tunnel: [_ w1118] -> _
          frame False {
          }
          frame True {
            n480 = call <vilib>:"G#Debugger_RunMethod.vi"("ClassPath"=w1120, "MethodName"="StartExternalCreateProcess.vi" ("name or relative path"), "ClassPrefix"=w1119, "error in (no error)"=w1122) -> ("Error?"=w1118:bool, "error out"=w1121:errorcluster)  [unwired: 13 in, 1 out]
          }
        }
        n481 = property on="External Create Process Running" class="Bool (strict)"("Value"=w1116) -> ()  [unwired: 2 in, 2 out]
        n482 = Generate User Event(user event=w1111, event data cluster="Clear" ("event data"), error in=w1113) -> (error out=w1114:errorcluster)  [unwired: 1 in, 1 out]
      }
      event "Destroy": Value Change {
        n483 = event-data() -> ()  [unwired: 1 in, 1 out]
        n484 = property class="Tree (strict)"(reference=w1128, error in=w1131) -> (error out=w1130:errorcluster, "Value"=w1127:string)  [unwired: 1 out]
        n485 = Unbundle By Name(w1125) -> ("ClassInfoDvr"=w1126:refnum<data-value>)
        n486 = disable-structure shown="Enabled" {
          disable-tunnel: w1130 -> [w1139 w1161]
          disable-tunnel: [w1135 w1161] -> w1129
          disable-tunnel: w1128 -> [w1134 _]
          disable-tunnel: w1127 -> [w1133 _]
          disable-tunnel: w1126 -> [w1132 _]
          frame Disabled {
            n487 = call <vilib>:"G#Debugger_GetObjectFromTag.vi"("Objects dvr"=w1132, "Tag"=w1133, "error in (no error)"=w1139) -> ("Ref"=w1136:refnum<class "G#Object.lvclass">, "Found"=w1137:bool, "error out"=w1138:errorcluster)  [unwired: 14 in]
            n488 = case shown="True" w1137 {
              tunnel: w1138 -> [w1140 w1146]
              tunnel: w1136 -> [_ w1148]
              tunnel: [w1140 w1147] -> w1135
              tunnel: w1134 -> [_ w1145]
              tunnel: w1133 -> [_ w1144]
              frame False {
              }
              frame True {
                w1150 = TRUE  # Simple Info
                n489 = call <vilib>:"G#Debugger_NavigateToPreviousTreeItem.vi"("Tree"=w1145, "Tag"=w1144, "error in (no error)"=w1146) -> ("error out"=w1143:errorcluster)  [unwired: 16 in]
                n490 = call <vilib>:"G#Object_SendUserEvent.vi"("text"="Debugger killed object!" ("Text"), "error in (no error)"=w1143) -> ("error out"=w1142:errorcluster)  [unwired: 16 in, 1 out]
                n491 = call-dynamic "GetObjectStatus.vi"("reference in"=w1148, "simple info (F)"=w1150, "error in (no error)"=w1142) -> ("# of users?"=w1149:i32, "error out"=w1151:errorcluster)  [unwired: 5 in, 10 out]
                n492 = for {
                  N: w1149 -> [_]
                  tunnel: [w1152] -> w1147
                  tunnel: w1151 -> [w1155]
                  tunnel: w1148 -> [w1154]
                  # "Loop users"
                  n493 = call-dynamic "NotARefNum.vi"("reference in"=w1154) -> ("not a refnum?"=w1153:bool)  [unwired: 1 in, 1 out]
                  n494 = case shown="False" w1153 {
                    tunnel: [w1157 w1160] -> w1152
                    tunnel: w1155 -> [w1159 w1160]
                    tunnel: w1154 -> [w1158 _]
                    frame False {
                      n495 = call-dynamic "Destroy.vi"("reference in"=w1158, "error in (no error)"=w1159) -> ("error out"=w1156:errorcluster)  [unwired: 16 in, 1 out]
                      n496 = call <vilib>:"Clear Errors.vi"("error in (no error)"=w1156) -> ("error out"=w1157:errorcluster)  [unwired: 5 in, 1 out]
                    }
                    frame True {
                    }
                  }
                }
              }
            }
          }
          frame Enabled {
          }
        }
      }
      event "Save": Value Change {
        n497 = event-data() -> ()  [unwired: 1 in, 1 out]
        n498 = property on="Trace" class="Str"() -> ("Value"=w1165:string)  [unwired: 2 in, 2 out]
        n499 = Write to Text File(text=w1165, error in=w1166) -> (error out=w1164:errorcluster)  [unwired: 2 in, 2 out]
        n500 = call <vilib>:"Clear Errors.vi"("error in (no error)"=w1164) -> ("error out"=w1163:errorcluster)  [unwired: 5 in, 1 out]
      }
      event "Enable Active Debug": Value Change {
        n501 = event-data() -> ("NewVal"=w1168:bool)  [unwired: 1 in]
        n502 = disable-structure shown="Enabled" {
          disable-tunnel: w1173 -> [w1182 _]
          disable-tunnel: w1172 -> [w1181 w1217]
          disable-tunnel: [w1180 w1217] -> w1171
          disable-tunnel: w1170 -> [w1179 _]
          disable-tunnel: w1169 -> [w1178 _]
          disable-tunnel: w1168 -> [w1174 _]
          frame Disabled {
            n503 = Select(t="Debugger enabled active debug!" ("Text"), s=w1174, f="Debugger disabled active debug!" ("Text")) -> (s? t:f=w1185:string)
            n504 = call <vilib>:"G#Object_SendUserEvent.vi"("text"=w1185, "error in (no error)"=w1181) -> ("error out"=w1177:errorcluster)  [unwired: 16 in, 1 out]
            n505 = call <vilib>:"G#Object_EnableDebug.vi"("set (F)"=TRUE, "debug enable (F)"=w1174, "error in (no error)"=w1177) -> ("error out"=w1176:errorcluster)  [unwired: 14 in, 2 out]
            n506 = case shown="True" w1174 {
              tunnel: w1176 -> [w1196 w1204]
              tunnel: [w1198 w1206] -> w1180
              tunnel: w1182 -> [w1197 w1205]
              tunnel: w1179 -> [w1187 w1203]
              tunnel: w1178 -> [_ w1200]
              frame False {
                n507 = Unbundle By Name(w1187) -> ("Front Panel"=w1186:refnum<vi>)
                n508 = call <vilib>:"G#Debugger_CachedObject.vi"("cached object"=refnum<class "G#Object.lvclass"> refnum, "error in (no error)"=w1196, "set"=TRUE) -> ("error out"=w1195:errorcluster)  [unwired: 14 in, 2 out]
                n509 = property on="Cached Reference Class Name" class="Str"("Value"="") -> ()  [unwired: 2 in, 2 out]
                n510 = call <vilib>:"GarbageCollector.vi"("error in (no error)"=w1195) -> ("error out"=w1189:errorcluster)  [unwired: 16 in, 2 out]
                n511 = property on="CachedObjId" class="DigNum (strict)"("Value"=u32 0 ("CachedObjId")) -> ()  [unwired: 2 in, 2 out]
                n512 = call "Empty Picture"() -> ("empty picture"=w1190:picture)
                n513 = invoke on="Method VI Panel" class="SubPanel" method="Remove VI"(error in=w1189) -> (error out=w1188:errorcluster)  [unwired: 2 in, 2 out]
                n514 = property on="Icon" class="Pict"("Value"=w1190) -> ()  [unwired: 2 in, 2 out]
                n515 = call <vilib>:"G#Debugger_ClearTree.vi"("Front Panel"=w1186, "Tree"=w1197, "error in (no error)"=w1188) -> ("error out"=w1198:errorcluster)  [unwired: 16 in]
              }
              frame True {
                n516 = Unbundle By Name(w1203) -> ("Front Panel"=w1199:refnum<vi>, "Active Project"=w1202:refnum<vi>)
                n517 = Not A Number/Path/Refnum?(number/path/refnum=w1202) -> (NaN/Path/Refnum?=w1201:bool)
                n518 = case shown="True" w1201 {
                  tunnel: [w1212 w1216] -> w1206
                  tunnel: w1205 -> [w1211 _]
                  tunnel: w1204 -> [w1209 w1216]
                  tunnel: w1202 -> [w1208 _]
                  tunnel: w1200 -> [_ w1215]
                  tunnel: w1199 -> [w1207 _]
                  frame False {
                    n519 = call <vilib>:"G#Object_StartExternalCreateProcess.vi"("error in (no error)"=w1209) -> ("error out"=w1210:errorcluster)  [unwired: 18 in]
                    n520 = call <vilib>:"G#Debugger_PopulateActiveDebugTree.vi"("Front Panel"=w1207, "Tree"=w1211, "Active Project"=w1208, "error in (no error)"=w1210) -> ("error out"=w1212:errorcluster)  [unwired: 15 in]
                  }
                  frame True {
                    (unwired) "%s not valid anymore!"
                    n521 = Format Into String(w1215) -> (resulting string=w1214:string)  [unwired: 3 in, 1 out]
                    n522 = property on="Enable Active Debug" class="Bool (strict)"("Value"=FALSE ("Enable Active Debug")) -> ()  [unwired: 2 in, 2 out]
                    n523 = One Button Dialog(message=w1214) -> ()  [unwired: 1 in, 1 out]
                  }
                }
              }
            }
          }
          frame Enabled {
          }
        }
      }
      event "Window Transparency": Value Change {
        # "#ToDo"
        n524 = event-data() -> ()  [unwired: 1 in, 1 out]
        n525 = Not Equal To 0?(x="Window Transparency") -> (x != 0?=w1219:bool)
        n526 = control-ref of="This VI"() -> (w1223:refnum<vi>)
        n527 = property class="VI"(reference=w1223, error in=w1222, "FP:Transparency"="Window Transparency", "FP:RunTransparently"=w1219) -> (error out=w1221:errorcluster)  [unwired: 1 out]
      }
      event "Window Behaviour": Value Change {
        n528 = event-data() -> ()  [unwired: 1 in, 5 out]
        n529 = Select(t=T10."Floating" ("Front Panel Window:Behavior"), s="Window Behaviour", f=T10."Default" ("Front Panel Window:Behavior")) -> (s? t:f=w1225:T10)
        n530 = property class="VI"(error in=w1230, "FP.Behavior"=w1225) -> (error out=w1229:errorcluster)  [unwired: 1 in, 1 out]
      }
      event "External Create Process Running": Value Change {
        n531 = event-data() -> ()  [unwired: 1 in, 1 out]
        n532 = Unbundle By Name(w1232) -> ("Path"=w1231:path)
        n533 = case shown="True" "External Create Process Running" {
          tunnel: w1236 -> [w1240 w1244]
          tunnel: [w1239 w1243] -> w1235
          tunnel: w1233 -> [w1238 w1245]
          tunnel: w1231 -> [w1237 w1242]
          frame False {
            n534 = call <vilib>:"G#Debugger_RunMethod.vi"("ClassPath"=w1237, "MethodName"="StopExternalCreateProcess.vi" ("name or relative path"), "ClassPrefix"=w1238, "error in (no error)"=w1240) -> ("error out"=w1239:errorcluster)  [unwired: 13 in, 2 out]
          }
          frame True {
            n535 = call <vilib>:"G#Debugger_RunMethod.vi"("ClassPath"=w1242, "MethodName"="StartExternalCreateProcess.vi" ("name or relative path"), "ClassPrefix"=w1245, "error in (no error)"=w1244) -> ("error out"=w1243:errorcluster)  [unwired: 13 in, 2 out]
          }
        }
      }
      event "Help": Value Change {
        n536 = event-data() -> ()  [unwired: 1 in, 5 out]
        n537 = property class="App"() -> ("OS.Name"=w1248:string, "OS.Version"=w1249:string)  [unwired: 2 in, 2 out]
        n538 = case shown="\"Windows\"..\"Windowt\"" w1248 {
          tunnel: w1249 -> [_ _]
          frame Default {
            n539 = call-poly <vilib>:"Open URL in Default Browser.vi"("URL"="http://www.addq.se/document/GsharpOnlineManual.htm" ("message")) -> ()  [unwired: 5 in, 2 out]
          }
          frame "Windows".."Windowt" {
            w1259 = TRUE  # run minimized? (F)
            w1260 = FALSE  # wait until completion? (T)
            n540 = VI Library() -> (path=w1258:path)
            n541 = Strip Path(path=w1258) -> (stripped path=w1257:path)  [unwired: 1 out]
            n542 = Build Path(base path=w1257, name or relative path="help") -> (appended path=w1255:path)
            n543 = Build Path(base path=w1255, name or relative path="_AddQ") -> (appended path=w1253:path)
            n544 = call <vilib>:"System Exec.vi"("run minimized? (F)"=w1259, "wait until completion? (T)"=w1260, "working directory"=w1253, "command line"="cmd /c hh.exe \"Gsharp.chm::GsharpDebugger.htm\"") -> ()  [unwired: 4 in, 4 out]
          }
        }
      }
      event "Filter Expression": Value Change {
        n545 = event-data() -> ("NewVal"=w1270:string)  [unwired: 1 in]
        n546 = Unbundle By Name(w1264) -> ("Path"=w1263:path)
        n547 = Format Into String(format string="Changed filter expression to '%s'!" ("text"), w1270) -> (resulting string=w1267:string)  [unwired: 2 in, 1 out]
        n548 = To Variant(anything=w1267) -> (Variant=w1268:variant)
        n549 = Build Array(w1268) -> (w1261:variant[])
        n550 = call <vilib>:"G#Debugger_RunMethod.vi"("ClassPath"=w1263, "MethodName"="SendUserEvent.vi" ("name or relative path"), "ClassPrefix"=w1262, "error in (no error)"=w1266, "ControlValue"=w1261) -> ("error out"=w1265:errorcluster)  [unwired: 12 in, 2 out]
      }
      event "Highlight Aggregates?": Value Change {
        n551 = event-data() -> ("NewVal"=w1275:bool)  [unwired: 1 in]
        n552 = case shown="False" w1275 {
          tunnel: w1277 -> [w1285 w1288]
          tunnel: w1276 -> [w1284 _]
          tunnel: [w1280 w1289] -> w1274
          tunnel: w1273 -> [w1279 w1287]
          frame False {
            # "redraw FP"
            n553 = Unbundle By Name(w1279) -> ("Front Panel"=w1278:refnum<vi>)
            n554 = call <vilib>:"G#Debugger_Highlight.vi"("Tree"=w1284, "error in (no error)"=w1285) -> ("error out"=w1281:errorcluster)  [unwired: 17 in]
            n555 = property class="Pnl"(reference=w1278, error in=w1281, "DeferPanUpdts"=FALSE ("Defer Panel Updates"), "DeferPanUpdts"=TRUE ("Defer Panel Updates")) -> (error out=w1280:errorcluster)  [unwired: 1 out]
          }
          frame True {
            n556 = Unbundle By Name(w1287) -> ("CloneUIevent"=w1286:refnum<user-event>)
            n557 = Generate User Event(user event=w1286, event data cluster="Highlight aggregates" ("event data"), error in=w1288) -> (error out=w1289:errorcluster)  [unwired: 1 in, 1 out]
          }
        }
      }
    }
    n558 = case shown="Error" w72 {
      selector: w72 -> [w87 w92]
      tunnel: [w87 w92] -> w73
      tunnel: w71 -> [_ w90]
      tunnel: [_ w88] -> _
      frame No Error {
      }
      frame Error {
        n559 = Unbundle By Name(w90) -> ("CloneUIevent"=w89:refnum<user-event>)
        n560 = Generate User Event(user event=w89, event data cluster="Exit" ("event data")) -> (error out=w88:errorcluster)  [unwired: 2 in, 1 out]
      }
    }
  }
  n561 = disable-structure shown="Disabled" {
    frame Disabled {
    }
    frame Enabled {
    }
  }
  n562 = Unregister For Events(event registration refnum=w61, error in=w62) -> (error out=w1:errorcluster)
  n563 = Unbundle By Name(w14) -> ("Active Project"=w20:refnum<vi>, "Front Panel"=w16:refnum<vi>, "CloneUIevent"=w24:refnum<user-event>, "ClassInfoDvr"=w25:refnum<data-value>, "sub panel dvr"=w26:refnum<data-value>)
  n564 = flat-sequence {
    tunnel: [errorcluster {"status"=FALSE, "code"=0, "source"=""} ("error in (no error)")] -> w2
    tunnel: w1 -> [w1291]
    tunnel: [w1291] -> w15
    frame #0 {
    }
  }
  n565 = Delete Data Value Reference(data value reference=w26, error in=w2) -> (data value=w31:T4, error out=w30:errorcluster)
  n566 = Unbundle By Name(w31) -> ("vi reference"=w27:refnum<vi>)
  n567 = Not A Number/Path/Refnum?(number/path/refnum=w27) -> (NaN/Path/Refnum?=w29:bool)
  n568 = case shown="False" w29 {
    tunnel: w30 -> [w1295 w1296]
    tunnel: [w1294 w1296] -> w28
    tunnel: w27 -> [w1293 _]
    frame False {
      n569 = Close Reference(reference=w1293, error in (no error)=w1295) -> (error out=w1294:errorcluster)
    }
    frame True {
    }
  }
  n570 = Delete Data Value Reference(data value reference=w25, error in=w28) -> (error out=w23:errorcluster)  [unwired: 1 out]
  n571 = disable-structure shown="Disabled" {
    disable-tunnel: w23 -> [w1307 _]
    disable-tunnel: [w1302 _] -> w22
    frame Disabled {
      # "If debugger created the\nevent-> kill it"
      n572 = Call Chain() -> (call chain=w1301:string[])
      n573 = Delete From Array(array=w1301) -> (deleted portion=w1300:string)  [unwired: 2 in, 1 out]
      n574 = call <vilib>:"G#Object_GetEvent.vi"("create if needed (T)"=FALSE ("create if needed"), "error in (no error)"=w1307) -> ("G# event"=w1303:refnum<user-event>, "valid"=w1298:bool, "event owner"=w1299:string, "error out"=w1305:errorcluster)  [unwired: 13 in, 1 out]
      n575 = Equal?(x=w1299, y=w1300) -> (x = y?=w1297:bool)
      n576 = And(x=w1298, y=w1297) -> (x .and. y?=w1304:bool)
      n577 = case shown="True" w1304 {
        tunnel: w1305 -> [w1308 w1311]
        tunnel: w1303 -> [_ w1310]
        tunnel: [w1308 w1309] -> w1302
        frame False {
        }
        frame True {
          n578 = Destroy User Event(user event=w1310, error in=w1311) -> (error out=w1309:errorcluster)
        }
      }
    }
    frame Enabled {
    }
  }
  n579 = Destroy User Event(user event=w24, error in=w22) -> (error out=w18:errorcluster)
  n580 = Close Reference(reference=w16, error in (no error)=w18) -> (error out=w17:errorcluster)
  n581 = Not A Number/Path/Refnum?(number/path/refnum=w20) -> (NaN/Path/Refnum?=w21:bool)
  n582 = case shown="False" w21 {
    tunnel: w17 -> [w1314 w1315]
    tunnel: [w1313 w1315] -> w19
    tunnel: w20 -> [w1312 _]
    frame False {
      n583 = Close Reference(reference=w1312, error in (no error)=w1314) -> (error out=w1313:errorcluster)
    }
    frame True {
    }
  }
  n584 = Merge Errors(w15, w19) -> (w12:errorcluster)
  n585 = case shown="Error" w12 {
    selector: w12 -> [w1316 w1318]
    tunnel: [w1316 _] -> w11
    frame No Error {
    }
    frame Error {
      n586 = Unbundle By Name(w1318) -> ("source"=w1317:string)
      n587 = One Button Dialog(message=w1317) -> ()  [unwired: 1 in, 1 out]
    }
  }
  n588 = invoke class="VI" method="FP.Close"(error in=w11) -> ()  [unwired: 2 in, 3 out]
